vi "VI Interference Konfig.vi"() -> ()   [LabVIEW 2020, in "EPA 1065.lvlib" / "HovaCAL Interference verificaton.lvlib"]
uses:
  HovaCAL Interference verificaton.lvlib
  Tabelle.ctl
  TestKonfig.ctl
  TestKonfig H2O.ctl
  Modus.ctl
  Linearisierung V2/SpanEinstellungen/Einheit.ctl
  Linearisierung V2/Gasteiler/Stufen Tabelle 10 Stufen.ctl
  Linearisierung V2/Gasteiler/HovaCAL_Interface/Controls/Flow Einstellung.ctl
  Linearisierung V2/Gasteiler/HovaCAL_Interface/Controls/Temp Sollwerte Anzeige.ctl
  TestKonfig Interferents.ctl
  MFCAuswahl.ctl
  Seiten/System Einstellungen V2/Gasflasche Auswahl.ctl
  TestSetting.ctl
  Seiten/System Einstellungen V2/Analysatoren.ctl
  Visualisierungs Elemente/String - Ausgabefeld.ctl
  Visualisierungs Elemente/Button.ctl
  Tabelle Referenz.ctl
  Linearisierung V2/Gasteiler/HovaCAL_Interface/Controls/Pumpe Status Anzeige.ctl
  Linearisierung V2/Gasteiler/HovaCAL_Interface/Controls/Temp Ausgang Anzeige.ctl
  Linearisierung V2/Gasteiler/Gasteiler Fehler.ctl
  Linearisierung V2/Gasteiler/HovaCAL_Interface/Controls/Flow Anzeige.ctl
  Linearisierung V2/Gasteiler/HovaCAL_Interface/Controls/MFC Output plus Input Output Concentrations.ctl
  Sprachverwaltung/FGV Aktion Tabelle zerlegen.ctl
  Linearisierung V2/Gasteiler/Aktionen FGV Gasteiler Daten.ctl
  Aktion FGV Interference.ctl
  Aktion Test.ctl
  Allgemeine VIs/Aktion Test Status.ctl
  Allgemeine VIs/Aktion Wertaenderung Gasliste.ctl
  Linearisierung V2/GasteilerType.ctl
  Linearisierung V2/Gasteiler/HovaCAL_Interface/Kommunikation/Aktion_FGV_HovaCAL_Interface_GetData.ctl
  Linearisierung V2/Gasteiler/HovaCAL_Interface/Kommunikation/Aktion_FGV_HovaCAL_Interface_SetData.ctl
  Linearisierung V2/Aktion FGV Stoerungen sammeln und auswerten.ctl
  Linearisierung V2/LIN ErrorCluster.ctl
  Linearisierung V2/Gasteiler/Gasteiler Stufen.ctl
  Visualisierungs Elemente/String - Eingabefeld.ctl
  Aktion Index uebersetzten.ctl
  Allgemein/allgemeine Sub-VIs.lvlib
  Seiten/FT-IR/FT-IR.lvlib
  Sprachverwaltung/Sprachverwaltung.lvlib
  Linearisierung V2/Protokoll/Protokoll.lvlib
  EPA 1065.lvlib
  Seiten/System Einstellungen V2/System Einstellungen V2.lvlib
  Linearisierung V2/Gasteiler/HovaCAL_Interface/Kommunikation/Aktion_FGV_HovaCAL_Interface_Kommandos.ctl
  Linearisierung V2/Gasteiler/HovaCAL_Interface/Kommunikation/Kommunikation.lvlib
  Linearisierung V2/Gasteiler/Gasteiler.lvlib
  Linearisierung V2/Linearisierung v2.lvlib
  Linearisierung V2/Gasteiler/HovaCAL_Interface/HovaCAL_Interface.lvlib
  Linearisierung V2/SpanEinstellungen/SpanEinstellungen.lvlib
  Linearisierung V2/Gasteiler/HovaCAL_Interface/Controls/Controls.lvlib
panel:
  in  "Graph löschen":bool caption="Test Start"
  out "Graph PDF":waveform(dbl)[](graph) caption="Graph"
  in  "Daten löschen":bool caption="Test Start"
  in  "Save to file":bool caption="PDF erstellen"
  in  "Speichern":bool
  in  "Gasliste vergleichen":bool
  in  "Systemeinstellung":bool caption="Gasliste geändert"
  in  "Registerkarte":T1(tab)
  in  "TestSetting":T2
  in  "Abfragen":T4
  in  "Anforderung":T4
  in  "TestKonfig":T5={"TestKonfig H2O"={"Modus"=0, "Komponente:"=0, "Eingangs Konzentration:"=0.0, "Einheit"=enum."ppm", "Anzahl Stufen"=0.0, "Zeitdauer Stufen"=0.0, "Max Fehler"=1.0, "zusätzliche Zeitdauer Erster Punkt"=60.0, "Punkte umkehren"=FALSE, "Stufen Tabelle"=[], "HovaCAL Flow Input Cluster"={"HovaCAL Flow Input Cluster"=0.0}, "HovaCAL Temperature"=[]}, "TestKonfig Interferent"={"MFC1"=enum."MFC 1", "Eingangs Konzentration MFC1"=0.0, "Einheit MFC1 Eingang"=enum."ppm", "Ausgangs Konzentration MFC1"=0.0, "Einheit MFC1 Ausgang"=enum."ppm", "MFC2"=0, "Referenz-Interferent:"=0, "Gasflaschen Nr MFC2"="", "Accuracy MFC2"="", "Eingangs Konzentration MFC2"=0.0, "Einheit MFC2 Eingang"=enum."ppm", "Ausgangs Konzentration MFC2"=0.0, "Einheit MFC2 Ausgang"=enum."ppm", "MFC3"=1, "Kontroll-Interferent:"=0, "Gasflaschen Nr MFC3"="", "Accuracy MFC3"="", "Eingangs Konzentration MFC3"=0.0, "Einheit MFC3 Eingang"=enum."ppm", "Ausgangs Konzentration MFC3"=120.0, "Einheit MFC3 Ausgang"=enum."ppm", "Gasflasche MFC2"=0, "Gasflasche MFC3"=0}} {"TestKonfig H2O"."HovaCAL Temperature" format="%.2f"; "TestKonfig H2O"."HovaCAL Flow Input Cluster"."HovaCAL Flow Input Cluster" format="%.2f"; "TestKonfig H2O"."Eingangs Konzentration:" min=0.0; "TestKonfig H2O"."Komponente:" items=["H2O% (30) LP 191C", "H2Oppm (300000)"]; "TestKonfig H2O"."zusätzliche Zeitdauer Erster Punkt" min=60 step=1 format="%#_5g"; "TestKonfig H2O"."Zeitdauer Stufen" format="%#_5g"; "TestKonfig H2O"."Max Fehler" format="%#_5g"; "TestKonfig H2O"."Anzahl Stufen" format="%#_5g"; "TestKonfig H2O"."Modus" items=["Messen", "CG zu Entnahmestelle"]; "TestKonfig Interferent"."Gasflasche MFC3" items=["----"=10000, "IAG O2"=0, "IAG C2H2"=1, "IAG C2H4"=2, "IAG NH3 200"=3, "IAG NH3 2000"=4, "IAG NH3 3000"=5, "IAG CO 5%"=6, "IAG Propane 2%"=7, "IAG NO 1000"=8, "IAG SO2"=9, "IAG C3H6"=10, "IAG CO2"=11, "IAG CO"=12, "IAG N2O"=13, "IAG N2O 100"=14, "IAG NO2 1000"=15, "IAG NO2 100"=16, "IAG CH4"=17, "IAG Propane"=18, "Hansi"=19, "IAG MG"=20, "IAG NO 3000"=21, "CH42"=22]; "TestKonfig Interferent"."Gasflasche MFC2" items=["----"=10000, "IAG O2"=0, "IAG C2H2"=1, "IAG C2H4"=2, "IAG NH3 200"=3, "IAG NH3 2000"=4, "IAG NH3 3000"=5, "IAG CO 5%"=6, "IAG Propane 2%"=7, "IAG NO 1000"=8, "IAG SO2"=9, "IAG C3H6"=10, "IAG CO2"=11, "IAG CO"=12, "IAG N2O"=13, "IAG N2O 100"=14, "IAG NO2 1000"=15, "IAG NO2 100"=16, "IAG CH4"=17, "IAG Propane"=18, "Hansi"=19, "IAG MG"=20, "IAG NO 3000"=21, "CH42"=22]; "TestKonfig Interferent"."Eingangs Konzentration MFC1" min=0.0; "TestKonfig Interferent"."Ausgangs Konzentration MFC1" min=0.0; "TestKonfig Interferent"."MFC2" items=["MFC2", "MFC3"]; "TestKonfig Interferent"."MFC3" items=["MFC2", "MFC3"]; "TestKonfig Interferent"."Ausgangs Konzentration MFC3" min=0.0; "TestKonfig Interferent"."Eingangs Konzentration MFC3" min=0.0; "TestKonfig Interferent"."Ausgangs Konzentration MFC2" min=0.0; "TestKonfig Interferent"."Eingangs Konzentration MFC2" min=0.0; "TestKonfig Interferent"."Kontroll-Interferent:" items=["NO (3000) LP 191C", "NO2 (150) LP 191C (1of2)", "NO2 (2000) LP 191C (2of2)", "N2O (300) LP 191C (1of2)", "NH3 (300) LP 191C (1of2)", "NH3 (900,3000) LP 191C (2of2)", "HNCO (400) 191C", "H2O% (30) LP 191C", "Formaldehyde (70,500) LP 191C", "CO2 low% (4) LP 191C (2of2)", "CO2% (20) LP 191C (1of2)", "CO (700) LP 191C (1of3)", "CO% (1) LP 191C (2of3)", "Propylene (1000) LP 191C", "Aromatic HC C7 (500) LP 191C", "Ethylene (1000) LP 191C", "CH4 (250) LP 191C (1of2)", "CH4 (5000) LP 191C (2of2)", "Ethane (1000) LP 191C", "Acetylene (1000) LP 191C", "HNO2 (20) 191C", "MeOH (1000) 191C", "CO% (10) LP 191C (3of3)", "Formic Acid (100) 191C", "SO2 (500) LP 191C", "Acetaldehyde (1000) LP 191C", "COS (100) LP 191C", "1,3 butadiene (100) LP 191C", "Oil as Octane (200) LP 191C", "N2O (1000) LP 191C (2of2)", "Propane (200) LP 191C", "NO2 autorange (2000)", "CO autorange (100000)", "CH4 autorange (5000)", "NH3 autorange (3000)", "NOx autorange (3000)", "HCD (10000)", "NMHCD (10000)", "CO2% autorange (20)", "H2Oppm (300000)", "N2O autorange (1000)", "NMNEHCD (3000)", "Temp. Messzelle", "Druck Messzelle", "sBeam@2500", "Temp. HL zu FT-IR", "Temp. HL Extern SP1", "Austrittstemp. FT-IR", "Temp. Schaltschrank", "Konstant 0", "Konstant 50", "Konstant 100", "AK DUMMY"]; "TestKonfig Interferent"."Referenz-Interferent:" items=["NO (3000) LP 191C", "NO2 (150) LP 191C (1of2)", "NO2 (2000) LP 191C (2of2)", "N2O (300) LP 191C (1of2)", "NH3 (300) LP 191C (1of2)", "NH3 (900,3000) LP 191C (2of2)", "HNCO (400) 191C", "H2O% (30) LP 191C", "Formaldehyde (70,500) LP 191C", "CO2 low% (4) LP 191C (2of2)", "CO2% (20) LP 191C (1of2)", "CO (700) LP 191C (1of3)", "CO% (1) LP 191C (2of3)", "Propylene (1000) LP 191C", "Aromatic HC C7 (500) LP 191C", "Ethylene (1000) LP 191C", "CH4 (250) LP 191C (1of2)", "CH4 (5000) LP 191C (2of2)", "Ethane (1000) LP 191C", "Acetylene (1000) LP 191C", "HNO2 (20) 191C", "MeOH (1000) 191C", "CO% (10) LP 191C (3of3)", "Formic Acid (100) 191C", "SO2 (500) LP 191C", "Acetaldehyde (1000) LP 191C", "COS (100) LP 191C", "1,3 butadiene (100) LP 191C", "Oil as Octane (200) LP 191C", "N2O (1000) LP 191C (2of2)", "Propane (200) LP 191C", "NO2 autorange (2000)", "CO autorange (100000)", "CH4 autorange (5000)", "NH3 autorange (3000)", "NOx autorange (3000)", "HCD (10000)", "NMHCD (10000)", "CO2% autorange (20)", "H2Oppm (300000)", "N2O autorange (1000)", "NMNEHCD (3000)", "Temp. Messzelle", "Druck Messzelle", "sBeam@2500", "Temp. HL zu FT-IR", "Temp. HL Extern SP1", "Austrittstemp. FT-IR", "Temp. Schaltschrank", "Konstant 0", "Konstant 50", "Konstant 100", "AK DUMMY"]}
  out "%":dbl caption="Komponente max Fehler:"
  out "Kontrollinterferentwert":dbl caption="ppm"
  out "Referenzinterferentwert":dbl caption="ppm"
  out "Komponentenwert":dbl caption="%"
  out "Testdauer":dbl caption="verbleibende Testdauer" format="%.1f"
  out "Referenzwert:":T15
  out "Referenzwert":dbl caption="ppm"
  out "Interferent 2:":T15 caption="Kontroll-Interferent:"
  out "Interferent 1:":T15 caption="Referenz-Interferent:"
  in  "Abbrechen":bool caption="Test Start"
  out "Graph":waveform(dbl)[](graph)
  out "Status":string caption="Zustand"
  in  "Test Start":bool
  out "Komponente 1S:":T15 caption="Komponente:"
  out "Störung Kommunikation":bool
  out "Kontroll Interferent":T16 caption="Kontroll-Interferent"
  out "Referenz Interferent":T17 caption="Referenz-Interferent"
  out "Komponente":T16
  in  "Print to PDF":bool caption="PDF erstellen"
  out "Error":T18
  out "Cluster.Temp Cluster":T19 caption="Temp Ausgang"
  out "Cluster.PumpModeGeneral-Cluster":T20 caption="Pumpe Status"
  out "MFC Output":T21 caption="Fluss gesamt" {"Actual Flow" format="%.2f"}
  out "Pumpe":T22 {"water conc set" format="%.2f"; "water conc out" format="%.2f"}
  out "MFC1 Output":T23 caption="MFC1" {"Input Concentration" format="%.2f"; "Output Setpoint" format="%.2f"; "flow expected" format="%.2f"; "flow actual" format="%.2f"; "output concentration dry" format="%.2f"; "output concentration" format="%.2f"}
  out "MFC2 Output":T23 caption="MFC2" {"Input Concentration" format="%.2f"; "Output Setpoint" format="%.2f"; "flow expected" format="%.2f"; "flow actual" format="%.2f"; "output concentration dry" format="%.2f"; "output concentration" format="%.2f"}
  out "MFC3 Output":T23 caption="MFC3" {"Input Concentration" format="%.2f"; "Output Setpoint" format="%.2f"; "flow expected" format="%.2f"; "flow actual" format="%.2f"; "output concentration dry" format="%.2f"; "output concentration" format="%.2f"}
  # "HovaCAL Querempfindlichkeitsnachweis"
  # "Allgemeine Einstellungen"
  # "Protokoll Einstellungen"
  # "Wasser"
  # "Stickstoff"
  # "Referenz-Interferent"
  # "Kontroll-Interferent"
  # "sec"
  # "%"
  # "sec"
  # "Test"
  # "sec"
  # "Ergebnis"
  # "%"
  # "%"
  # "l/min"
  # "l/min"
  # "l/min"
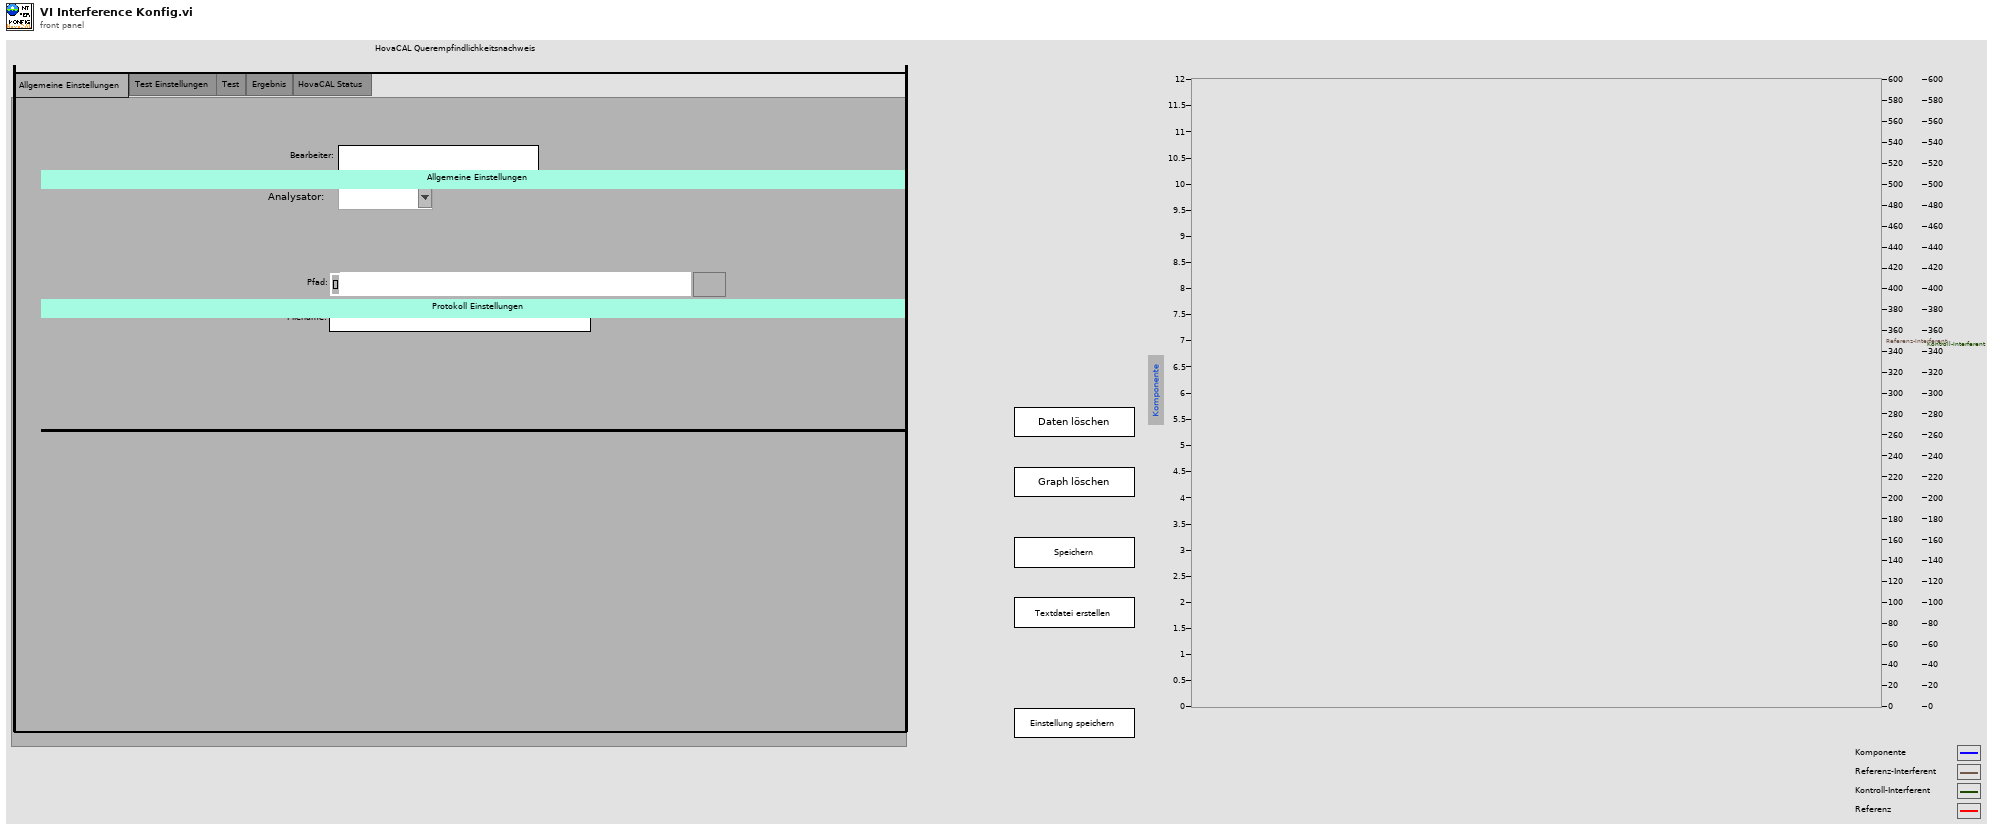
[diagram p1: front panel]
types:
  T1 = enum32{"General Settings", "Test Settings", "Test", "Result", "HovaCAL Status"}
  T2 = typedef "EPA 1065.lvlib/HovaCAL Interference verificaton.lvlib/TestSetting.ctl" = cluster{"Bearbeiter:":string, "Pfad:":path, "Textname:":string, "Analysator":T3}
  T3 = typedef "System Einstellungen V2.lvlib/Analysatoren.ctl" = string
  T4 = typedef "Button.ctl" = bool
  T5 = typedef "EPA 1065.lvlib/HovaCAL Interference verificaton.lvlib/TestKonfig.ctl" = cluster{"TestKonfig H2O":T6, "TestKonfig Interferent":T12}
  T6 = typedef "EPA 1065.lvlib/HovaCAL Interference verificaton.lvlib/TestKonfig H2O.ctl" = cluster{"Modus":T7, "Komponente:":u16, "Eingangs Konzentration:":dbl, "Einheit":T8, "Anzahl Stufen":sgl, "Zeitdauer Stufen":sgl, "Max Fehler":sgl, "zusätzliche Zeitdauer Erster Punkt":sgl, "Punkte umkehren":bool, "Stufen Tabelle":T9, "HovaCAL Flow Input Cluster":T10, "HovaCAL Temperature":T11}
  T7 = typedef "EPA 1065.lvlib/HovaCAL Interference verificaton.lvlib/Modus.ctl" = u16
  T8 = typedef "Linearisierung v2.lvlib/SpanEinstellungen.lvlib/Einheit.ctl" = enum16{"ppm", "%"}
  T9 = typedef "Linearisierung v2.lvlib/Gasteiler.lvlib/Stufen Tabelle 10 Stufen.ctl" = string[][]
  T10 = typedef "Linearisierung v2.lvlib/Gasteiler.lvlib/HovaCAL_Interface.lvlib/Controls.lvlib/Flow Einstellung.ctl" = cluster{"HovaCAL Flow Input Cluster":dbl}
  T11 = typedef "Linearisierung v2.lvlib/Gasteiler.lvlib/HovaCAL_Interface.lvlib/Controls.lvlib/Temp Sollwerte Anzeige.ctl" = dbl[]
  T12 = typedef "EPA 1065.lvlib/HovaCAL Interference verificaton.lvlib/TestKonfig Interferents.ctl" = cluster{"MFC1":enum16{"MFC 1"}, "Eingangs Konzentration MFC1":dbl, "Einheit MFC1 Eingang":T8, "Ausgangs Konzentration MFC1":dbl, "Einheit MFC1 Ausgang":T8, "MFC2":T13, "Referenz-Interferent:":u16, "Gasflaschen Nr MFC2":string, "Accuracy MFC2":string, "Eingangs Konzentration MFC2":dbl, "Einheit MFC2 Eingang":T8, "Ausgangs Konzentration MFC2":dbl, "Einheit MFC2 Ausgang":T8, "MFC3":T13, "Kontroll-Interferent:":u16, "Gasflaschen Nr MFC3":string, "Accuracy MFC3":string, "Eingangs Konzentration MFC3":dbl, "Einheit MFC3 Eingang":T8, "Ausgangs Konzentration MFC3":dbl, "Einheit MFC3 Ausgang":T8, "Gasflasche MFC2":T14, "Gasflasche MFC3":T14}
  T13 = typedef "EPA 1065.lvlib/HovaCAL Interference verificaton.lvlib/MFCAuswahl.ctl" = u16
  T14 = typedef "System Einstellungen V2.lvlib/Gasflasche Auswahl.ctl" = u16
  T15 = typedef "String - Ausgabefeld.ctl" = string
  T16 = typedef "EPA 1065.lvlib/HovaCAL Interference verificaton.lvlib/Tabelle.ctl" = string[][]
  T17 = typedef "EPA 1065.lvlib/HovaCAL Interference verificaton.lvlib/Tabelle Referenz.ctl" = string[][]
  T18 = typedef "Linearisierung v2.lvlib/Gasteiler.lvlib/Gasteiler Fehler.ctl" = cluster{"Pressure carrier gas":bool, "Pressure diluted gas":bool, "Outlet Pressure":bool, "SNOX before SAIR":bool}
  T19 = typedef "Linearisierung v2.lvlib/Gasteiler.lvlib/HovaCAL_Interface.lvlib/Controls.lvlib/Temp Ausgang Anzeige.ctl" = cluster{"temp 2":dbl, "temp":dbl, "humidity":dbl}[]
  T20 = typedef "Linearisierung v2.lvlib/Gasteiler.lvlib/HovaCAL_Interface.lvlib/Controls.lvlib/Pumpe Status Anzeige.ctl" = cluster{"running?":bool, "Speed":dbl[]}
  T21 = typedef "Linearisierung v2.lvlib/Gasteiler.lvlib/HovaCAL_Interface.lvlib/Controls.lvlib/Flow Anzeige.ctl" = cluster{"Actual Flow":dbl}
  T22 = cluster{"water conc set":dbl, "water conc out":dbl}
  T23 = typedef "Linearisierung v2.lvlib/Gasteiler.lvlib/HovaCAL_Interface.lvlib/Controls.lvlib/MFC Output plus Input Output Concentrations.ctl" = cluster{"Input Concentration":dbl, "Output Setpoint":dbl, "output concentration":dbl, "output concentration dry":dbl, "flow actual":dbl, "flow expected":dbl}
  T24 = typedef "EPA 1065.lvlib/HovaCAL Interference verificaton.lvlib/Aktion Test.ctl" = enum16{"Lesen", "ini", "ini-Warten-Stabil", "Warten-Stabil", "ini-warten-aufzeichnen", "Warten-Aufzeichnen", "aufzeichnen", "fertig", "spülen", "abbrechen"}
  T25 = typedef "EPA 1065.lvlib/HovaCAL Interference verificaton.lvlib/Aktion FGV Interference.ctl" = enum16{"Lesen", "TestKonfig", "TestSetting", "Einheiten", "Ergebnis", "Laden", "Tabelle", "Speichern", "löschen"}
  T26 = typedef "Linearisierung v2.lvlib/Gasteiler.lvlib/Aktionen FGV Gasteiler Daten.ctl" = enum16{"lesen", "Gasteiler Daten", "Seriellen Param.", "MB-Endwert", "laden", "speichern", "Anforderung", "TCP", "Aufzeichnung Start"}
  T27 = typedef "Sprachverwaltung.lvlib/FGV Aktion Tabelle zerlegen.ctl" = enum16{"laden", "vereinzeln", "speichern"}
  T28 = typedef "EPA 1065.lvlib/HovaCAL Interference verificaton.lvlib/Komponenten.ctl" = cluster{"Komponente":T15, "Komponente Index":i32, "Referenz Interferent":T15, "Refernz Interferent Index":i32, "Kontroll Interferent":T15, "Kontroll Interferent Index":i32, "Einheit Komponente":string, "Einheit Refernz Interferrent":string, "Einheit Kontroll Interferrent":string}
  T29 = typedef "Linearisierung v2.lvlib/Gasteiler.lvlib/HovaCAL_Interface.lvlib/Kommunikation.lvlib/Aktion_FGV_HovaCAL_Interface_GetData.ctl" = enum16{"lesen", "SystemInfo", "MFC Info", "actual Values", "Limits", "first contact", "reset after read"}
  T30 = enum8{"Enabled", "Disabled", "Disabled and Grayed Out"}
  T31 = typedef "EPA 1065.lvlib/Aktion Wertaenderung Gasliste.ctl" = enum16{"Init", "lesen", "Gasliste geändert", "ARN inaktiv", "LEAK inaktiv", "Interference 366 inaktiv", "T90 inaktiv", "Interference 375 inaktiv", "Chiller inaktiv", "FID O2 inaktiv", "FID Opti inaktiv", "Drift inaktiv", "Pre Test inaktiv", "LinV2 inaktiv", "HovaCAL Interference inaktiv"}
  T32 = typedef "EPA 1065.lvlib/Aktion Test Status.ctl" = enum16{"init", "lesen", "prüfen", "Interference 366", "Interference 375", "Chiller läuft", "Drift läuft", "Pre Test läuft", "FID Optimization läuft", "FID Interference läuft", "HovaCAL Interference", "LinV2"}
  T33 = typedef "Linearisierung v2.lvlib/Gasteiler.lvlib/HovaCAL_Interface.lvlib/Kommunikation.lvlib/Aktion_FGV_HovaCAL_Interface_SetData.ctl" = enum16{"lesen", "Konzentrationen", "Pumpen Parameter", "Pumpe Konzentration", "Pumpe run", "Temperaturen", "Fluss", "Limits", "init"}
  T34 = typedef "Linearisierung v2.lvlib/Gasteiler.lvlib/HovaCAL_Interface.lvlib/Kommunikation.lvlib/Aktion_FGV_HovaCAL_Interface_Kommandos.ctl" = enum16{"lesen", "verarbeiten", "hinzufügen", "on top", "init", "sammeln", "freigeben", "connected"}
  T35 = enum32{"General Settings", "Test Settings", "Test", "Result"}
  T36 = typedef "String - Eingabefeld.ctl" = string
  T37 = typedef "Linearisierung v2.lvlib/LIN ErrorCluster.ctl" = cluster{"Störung Kommunikation":bool, "Pressure carrier gas":bool, "Pressure diluted gas":bool, "Outlet Pressure":bool, "SNOX before SAIR":bool, "Störung Gasteiler":bool}
  T38 = typedef "Linearisierung v2.lvlib/Aktion FGV Stoerungen sammeln und auswerten.ctl" = enum16{"init", "lesen", "error", "prüfen", "reset error", "abbrechen", "fortsetzen", "neustart", "Bedientasten reset"}
  T39 = typedef "EPA 1065.lvlib/HovaCAL Interference verificaton.lvlib/Aktion Index uebersetzten.ctl" = enum16{"lesen", "schreiben", "auswerten", "Referenzwert", "KompIndex", "RefInterferIndex", "KontrInterfIndex"}
  T40 = enum16{"open", "replace", "create", "open or create", "replace or create", "replace or create with confirmation"}
  T41 = cluster{"first contact in":bool, "first actual values in ":bool}
  T42 = typedef "Linearisierung v2.lvlib/GasteilerType.ctl" = u16
  T43 = typedef "EPA 1065.lvlib/Aktive Tests Cluster.ctl" = cluster{"ANR läuft":bool, "T90 läuft":bool, "Leak läuft":bool, "Interference 366 läuft":bool, "Interference 375 läuft":bool, "Chiller läuft":bool, "FID Interference läuft":bool, "FID optimization läuft":bool, "Drift läuft":bool, "Pre-test läuft":bool, "HovaCAL Interference läuft":bool, "LinV2 läuft":bool}
  T44 = typedef "LVDateTimeRec.ctl" = cluster{"Sekundenbruchteil":dbl, "Sekunde":i32, "Minute":i32, "Stunde":i32, "Tag des Monats":i32, "Monat":i32, "Jahr":i32, "Wochentag":i32, "Tag des Jahres":i32, "DST":i32}
  T45 = cluster{"temp 2":dbl, "temp":dbl, "humidity":dbl}[]
  T46 = typedef "Linearisierung v2.lvlib/Gasteiler.lvlib/HovaCAL_Interface.lvlib/Controls.lvlib/Info Cluster.ctl" = cluster{"device":string, "version":string, "number of mfc":i32, "number of pumps":i32, "number of temp controllers":i32, "number of mfs":i32, "number of balances":i32}
  T47 = cluster{"HovaCAL Temperature":refnum<vi>, "Cluster.Temp Cluster":refnum<vi>, "Cluster.PumpModeGeneral-Cluster":refnum<vi>, refnum<vi>[]}
  T48 = typedef "Linearisierung v2.lvlib/Gasteiler.lvlib/Gasteiler Stufen.ctl" = u16
  T49 = typedef "Linearisierung v2.lvlib/Gasteiler.lvlib/Gasteiler Daten.ctl" = cluster{"Gasteiler":T36, "Gasteiler Stufen":T48, "Gasteiler Type":T42, "Konfig Gasteiler":T50, "Gasteiler Span Eingänge":u16}
  T50 = typedef "System Einstellungen V2.lvlib/Gasteiler Auswahl.ctl" = u16
  T51 = cluster{"Komponente:":u16, "Eingangs Konzentration:":dbl}[]
  T52 = cluster{"Komponente:":u16, "Eingangs Konzentration:":dbl}
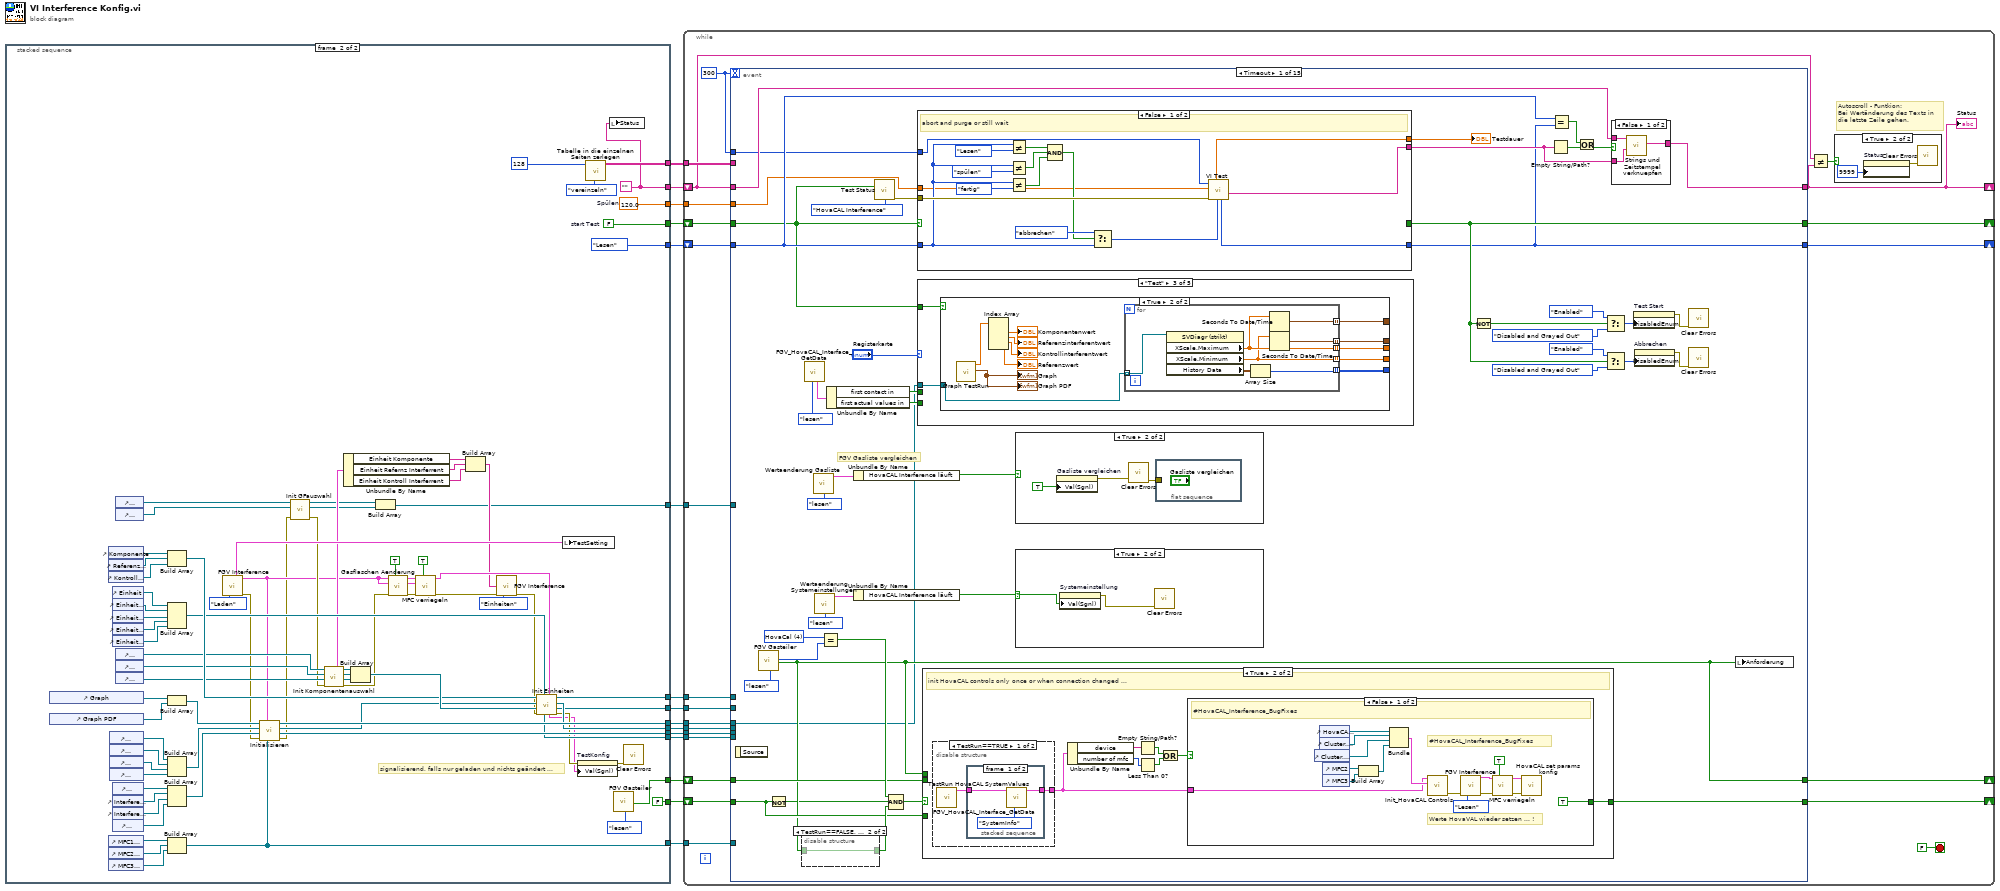
[diagram p0: block diagram]
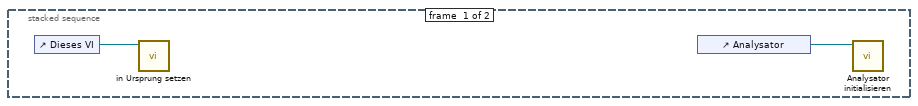
[diagram p2: hidden frame]
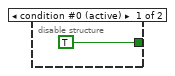
[diagram p3: hidden frame]
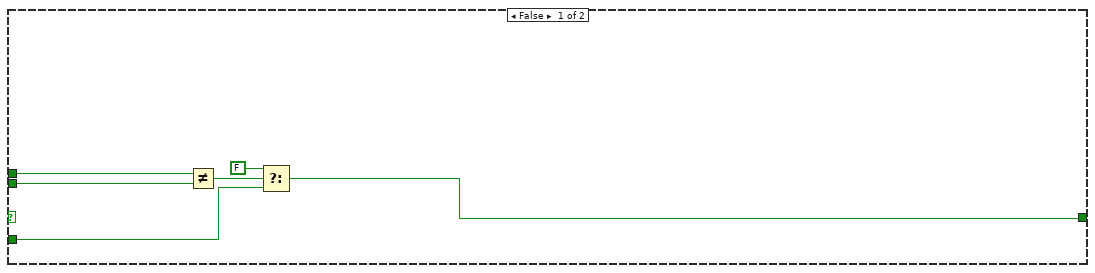
[diagram p4: hidden frame]
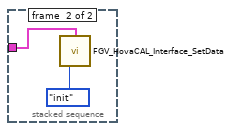
[diagram p6: hidden frame]
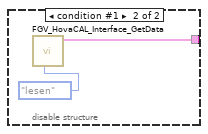
[diagram p7: hidden frame]
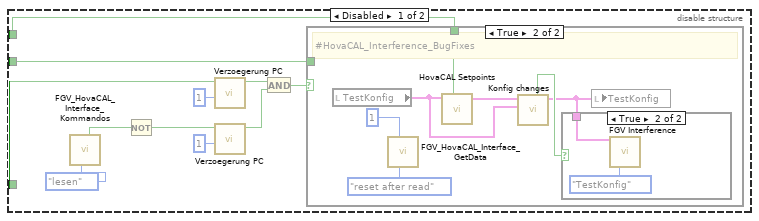
[diagram p12: hidden frame]
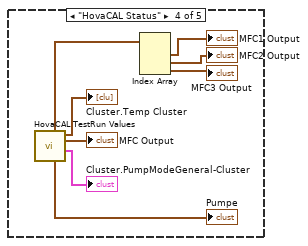
[diagram p16: hidden frame]
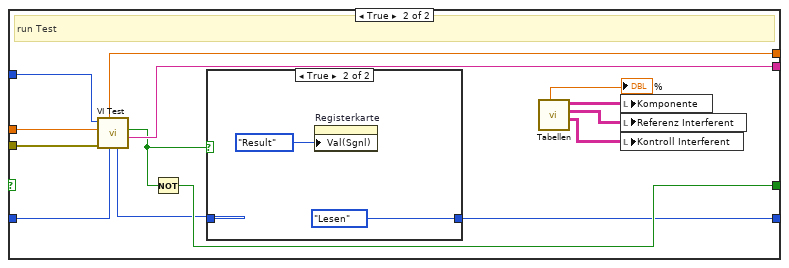
[diagram p18: hidden frame]
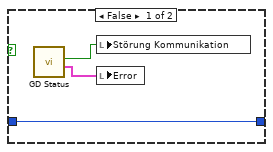
[diagram p19: hidden frame]
diagram:
  n1 = stacked-sequence {
    tunnel: [_ w97] -> w15
    tunnel: [_ w90] -> w14
    tunnel: [_ w87] -> w13
    tunnel: [_ w80] -> w12
    tunnel: [_ w86] -> w11
    tunnel: [_ w79] -> w10
    tunnel: [_ FALSE] -> w9
    tunnel: [_ w62] -> w8
    tunnel: [_ w69] -> w7
    tunnel: [_ w60] -> w6
    tunnel: [_ Aktion_Test."Lesen" ("Aktion")] -> w5
    tunnel: [_ w35] -> w4
    tunnel: [_ w26] -> w3
    tunnel: [_ w19] -> w2
    tunnel: [_ w18] -> w1
    frame #0 {
      n2 = control-ref of="Dieses VI"() -> (w16:refnum<vi>)
      n3 = call "in Ursprung setzen.vi"("VI Referenz"=w16) -> ()  [unwired: 10 in, 1 out]
      n4 = control-ref of="Analysator"() -> (w17:refnum<vi>)
      n5 = call "Analysator initialisieren.vi"("Referenz Analysator"=w17) -> ()  [unwired: 9 in, 2 out]
    }
    frame #1 {
      w18 = 120.0  # Spülen
      w35 = ""
      w90 = FALSE  # start Test
      # "signalisierend, falls nur geladen und nichts geändert ..."
      n6 = control-ref of="Graph"() -> (w88:refnum<vi>)
      n7 = control-ref of="Graph PDF"() -> (w75:refnum<vi>)
      n8 = control-ref of="Komponente"() -> (w73:refnum<vi>)
      n9 = control-ref of="Referenz Interferent"() -> (w72:refnum<vi>)
      n10 = control-ref of="Kontroll Interferent"() -> (w71:refnum<vi>)
      n11 = control-ref of="MFC1 Output"() -> (w22:refnum<vi>)
      n12 = control-ref of="MFC2 Output"() -> (w21:refnum<vi>)
      n13 = control-ref of="MFC3 Output"() -> (w20:refnum<vi>)
      n14 = control-ref of="Komponentenwert"() -> (w32:refnum<vi>)
      n15 = control-ref of="Referenzinterferentwert"() -> (w33:refnum<vi>)
      n16 = control-ref of="Kontrollinterferentwert"() -> (w34:refnum<vi>)
      n17 = control-ref of="Referenzwert"() -> (w77:refnum<vi>)
      n18 = control-ref of="Einheit"() -> (w68:refnum<vi>)
      n19 = control-ref of="Einheit MFC2 Eingang"() -> (w67:refnum<vi>)
      n20 = control-ref of="Einheit MFC2 Ausgang"() -> (w66:refnum<vi>)
      n21 = control-ref of="Einheit MFC3 Eingang"() -> (w65:refnum<vi>)
      n22 = control-ref of="Einheit MFC3 Ausgang"() -> (w64:refnum<vi>)
      n23 = control-ref of="Komponente 1S:"() -> (w89:refnum<vi>)
      n24 = control-ref of="Interferent 1:"() -> (w94:refnum<vi>)
      n25 = control-ref of="Interferent 2:"() -> (w95:refnum<vi>)
      n26 = control-ref of="Referenzwert:"() -> (w78:refnum<vi>)
      n27 = control-ref of="Gasflasche MFC2"() -> (w31:refnum<vi>)
      n28 = control-ref of="Gasflasche MFC3"() -> (w30:refnum<vi>)
      n29 = control-ref of="Komponente:"() -> (w49:refnum<vi>)
      n30 = control-ref of="Referenz-Interferent:"() -> (w48:refnum<vi>)
      n31 = control-ref of="Kontroll-Interferent:"() -> (w47:refnum<vi>)
      n32 = Build Array(w73, w72, w71) -> (w63:refnum<vi>[])
      n33 = Build Array(w68, w67, w66, w65, w64) -> (w61:refnum<vi>[])
      n34 = Build Array(w88, w75) -> (w76:refnum<vi>[])
      n35 = Build Array(w32, w33, w34, w77) -> (w93:refnum<vi>[])
      n36 = Build Array(w89, w94, w95, w78) -> (w92:refnum<vi>[])
      n37 = Build Array(w22, w21, w20) -> (w19:refnum<vi>[])
      n38 = call "FGV Interference.vi"("Aktion FGV Interference"=Aktion_FGV_Interference."Laden") -> ("TestSetting"=w58:T2, "TestKonfig"=w25:T5, "error out"=w24:errorcluster)  [unwired: 9 in, 3 out]
      n39 = call "Initialisieren.vi"("MFC Cluster Array"=w19, "TestKonfig (Eingang)"=w25, "Fehler (Eingang)"=w24, "Strings Array in"=w92, "Ergebnis  Array in"=w93, "Signalverlaufsdiagramm (Eingang)"=w76) -> ("Fehler (Ausgang)"=w23:errorcluster, "Strings Array out"=w86:refnum<vi>[], "Ergenis Arry out"=w81:refnum<vi>[], "Signalverlaufsdiagramm (Ausgang)"=w87:refnum<vi>[])  [unwired: 2 in]
      n40 = call "Init GFauswahl.vi"("Fehler (Eingang, kein Fehler)"=w23, "GF MFC3 (Eingang)"=w30, "GF MFC2 (Eingang)"=w31) -> ("Fehler (Ausgang)"=w29:errorcluster, "GF MFC3 (Ausgang)"=w27:refnum<vi>, "GF MFC2 (Ausgang)"=w28:refnum<vi>)  [unwired: 6 in]
      n41 = call "Init Komponentenauswahl.vi"("Fehler (Eingang, kein Fehler)"=w29, "Kontroll-Interferent: (Eingang)"=w47, "Refernz-Interferent: (Eingang)"=w48, "Komponente: (Eingang)"=w49) -> ("Fehler (Ausgang)"=w40:errorcluster, "Kontroll-Interferent: (Ausgang)"=w83:refnum<vi>, "Refernz-Interferent:  (Ausgang)"=w84:refnum<vi>, "Komponente: (Ausgang)"=w85:refnum<vi>, "Komponenten"=w41:T28)  [unwired: 3 in]
      n42 = Unbundle By Name(w41) -> ("Einheit Komponente"=w45:string, "Einheit Refernz Interferrent"=w44:string, "Einheit Kontroll Interferrent"=w43:string)
      n43 = Build Array(w85, w84, w83) -> (w82:refnum<vi>[])
      n44 = Build Array(w28, w27) -> (w26:refnum<vi>[])
      n45 = call "Gasflaschen Aenderung.vi"("init"=TRUE, "Fehler (Eingang, kein Fehler)"=w40, "TestKonfig alt"=w25, "TestKonfig (Eingang)"=w25) -> ("Fehler (Ausgang)"=w51:errorcluster, "TestKonfig alt out"=w52:T5, "TestKonfig (Ausgang)"=w53:T5)  [unwired: 5 in]
      n46 = call "MFC verriegeln.vi"("init"=TRUE, "Fehler (Eingang, kein Fehler)"=w51, "TestKonfig alt (Eingang)"=w52, "TestKonfig (Eingang)"=w53) -> ("Fehler (Ausgang)"=w39:errorcluster, "TestKonfig (Ausgang)"=w50:T5)  [unwired: 5 in, 1 out]
      n47 = Build Array(w45, w44, w43) -> (w42:string[])
      n48 = call "FGV Interference.vi"("Einheiten"=w42, "error in (no error)"=w39, "Aktion FGV Interference"=Aktion_FGV_Interference."Einheiten") -> ("error out"=w38:errorcluster)  [unwired: 7 in, 5 out]
      n49 = call "Init Einheiten.vi"("TestKonfig (Eingang)"=w50, "Units Array in"=w61, "Fehler (Eingang, kein Fehler)"=w38, "Komp. Auswahl Array"=w82, "Ergebnis Array in"=w81, "Table Array in"=w63) -> ("Fehler (Ausgang)"=w55:errorcluster, "Komp. Auswahl Array out"=w79:refnum<vi>[], "Ergebnis Array out"=w80:refnum<vi>[], "Table Array out"=w62:refnum<vi>[], "TestKonfig (Ausgang)"=w37:T5, "Units Array out"=w60:refnum<vi>[])
      n50 = local write "TestSetting"(w58) -> ()
      n51 = property on="TestKonfig" class="Cluster (strikt)"(error in=w55, "Val(Sgnl)"=w37) -> (error out=w59:errorcluster)  [unwired: 1 in, 1 out]
      n52 = call "Tabelle in die einzelnen Seiten zerlegen.vi"("Aktion"=FGV_Aktion_Tabelle_zerlegen."vereinzeln", "Index (Seite)"=128) -> ("Sprachliste"=w97:string[][])  [unwired: 7 in, 2 out]
      n53 = local write "Status"(w35) -> ()
      n54 = call "FGV Gasteiler.vi"("Aktionen"=Aktionen_FGV_Gasteiler_Daten."lesen") -> ("Anforderung"=w69:bool)  [unwired: 11 in, 7 out]
      n55 = call <vilib>:"Clear Errors.vi"("error in (no error)"=w59) -> ()  [unwired: 5 in, 2 out]
    }
  }
  n56 = while {
    shift-right: [w118] -> _
    shift-left: w14 -> [w119]
    shift-right: [w114] -> _
    shift-left: w4 -> [w116]
    tunnel: w15 -> [w117]
    shift-right: [w113] -> _
    shift-left: w5 -> [w112]
    tunnel: w13 -> [w111]
    tunnel: w12 -> [w110]
    tunnel: w11 -> [w109]
    tunnel: w10 -> [w108]
    shift-right: [w106] -> _
    shift-left: w9 -> [w107]
    tunnel: w8 -> [w105]
    shift-right: [w104] -> _
    shift-left: w7 -> [w103]
    tunnel: w6 -> [w102]
    tunnel: w3 -> [w100]
    tunnel: w2 -> [w99]
    tunnel: w1 -> [w98]
    stop <- FALSE stop-if-true
    w101 = 300
    # "Autoscroll - Funtkion:\nBei Wertänderung des Texts in \ndie letzte Zeile gehen."
    n57 = event shown="[0] Timeout" {
      selector: _ -> [_ _ _ _ _ _ _ _ _ _ _ _ _ _ _]
      dyn-events: _ -> [_ _ _ _ _ _ _ _ _ _ _ _ _ _ _]
      timeout: w101 -> [_ _ _ _ _ _ _ _ _ _ _ _ _ _ _]
      tunnel: [w165 w331 w355 w365 w385 w439 w478 w481 w558 w569 w592 w605 w628 w636 w642] -> w114
      tunnel: w116 -> [w164 w331 w355 w365 w385 w439 w478 _ w557 w569 w592 w605 w628 w636 w642]
      tunnel: w119 -> [w127 w330 w356 w362 w386 w441 w477 _ _ w571 w591 w604 w630 w638 w643]
      tunnel: [w145 w330 w356 w361 w386 w441 w477 w493 FALSE w571 w591 w604 w630 w638 w643] -> w118
      tunnel: w117 -> [_ _ _ w359 _ _ w443 w489 w554 _ _ _ _ _ _]
      tunnel: [w131 w329 w357 w364 w387 w440 w476 w491 w556 w570 w590 w603 w629 w637 w644] -> w113
      tunnel: w112 -> [w130 w329 w357 w364 w387 w440 w476 w490 w556 w570 w590 w603 w629 w637 w644]
      tunnel: w111 -> [w121 _ _ _ _ w426 _ w483 _ _ w578 _ _ w634 _]
      tunnel: w110 -> [_ _ _ _ _ w438 w451 w482 _ _ _ _ _ w633 _]
      tunnel: w109 -> [_ _ _ _ _ w437 _ _ _ _ _ _ _ _ _]
      tunnel: w108 -> [_ _ _ _ _ w436 w450 _ _ _ _ _ _ _ _]
      tunnel: w107 -> [w136 _ w332 w358 w381 w390 w442 w480 w547 w565 w572 w601 w626 w632 w639]
      tunnel: [w138 FALSE ("t") w332 w358 w381 w390 w442 w480 w547 w565 w572 w601 w626 w632 w639] -> w106
      tunnel: w105 -> [_ _ _ _ _ w415 w452 _ _ _ _ _ _ _ _]
      tunnel: [w134 w305 w354 w363 w382 w417 w475 w484 w548 w566 w576 w602 w627 w635 w641] -> w104
      tunnel: w103 -> [w135 w305 w354 w363 w382 w417 w475 w484 w548 w566 w576 w602 w627 w635 w641]
      tunnel: w102 -> [_ _ _ _ _ w416 w453 _ _ _ _ _ _ _ _]
      tunnel: w101 -> [w128 _ _ _ _ _ _ _ _ _ _ _ _ _ _]
      tunnel: w100 -> [_ _ _ w360 _ _ _ _ _ _ _ _ _ _ _]
      tunnel: w99 -> [_ _ _ _ _ w392 _ _ _ _ _ _ _ _ _]
      tunnel: w98 -> [w122 _ _ _ _ _ _ w479 _ _ _ _ _ _ _]
      event Timeout {
        w142 = T42 4 items=["LNI", "Analog-Display", "AVL GDU", "Horiba GDC", "HovaCal", "Horiba SGD 710C"] ("x")
        # "FGV Gasliste vergleichen"
        n58 = event-data() -> ()  [unwired: 1 in, 1 out]
        n59 = call "FGV Gasteiler.vi"("Aktionen"=Aktionen_FGV_Gasteiler_Daten."lesen") -> ("Gasteiler Type"=w141:T42, "Anforderung"=w134:bool)  [unwired: 11 in, 6 out]
        n60 = Not(x=w136) -> (.not. x?=w129:bool)
        n61 = disable-structure shown="TestRun==FALSE, Standard" {
          disable-tunnel: [TRUE w169] -> w137
          disable-tunnel: w134 -> [_ w169]
          frame condition #0 (active) {
          }
          frame condition #1 {
          }
        }
        n62 = call "FGV_HovaCAL_Interface_GetData.vi"("Aktion"=Aktion_FGV_HovaCAL_Interface_GetData."lesen") -> ("first flags out"=w126:T41)  [unwired: 6 in, 4 out]
        n63 = call "Wertaenderung Gasliste.vi"("Aktion"=Aktion_Wertaenderung_Gasliste."lesen") -> ("Tests"=w160:T43)  [unwired: 13 in, 1 out]
        n64 = call "Wertaenderung Systemeinstellungen.vi"("Aktion"=Aktion_Wertaenderung_Gasliste."lesen") -> ("Tests"=w156:T43)  [unwired: 13 in, 1 out]
        n65 = Equal?(x=w142, y=w141) -> (x = y?=w139:bool)
        n66 = Unbundle By Name(w126) -> ("first contact in"=w123:bool, "first actual values in"=w124:bool)
        n67 = Unbundle By Name(w160) -> ("HovaCAL Interference läuft"=w159:bool)
        n68 = Unbundle By Name(w156) -> ("HovaCAL Interference läuft"=w157:bool)
        n69 = call "Test Status.vi"("HovaCAL Interference läuft"=w127, "Aktion"=Aktion_Test_Status."HovaCAL Interference") -> ("error out"=w155:errorcluster)  [unwired: 10 in, 3 out]
        n70 = Compound Arithmetic op=AND ("Mehrfacharithmetik")(w139, w129, w137) -> (w140:bool)
        n71 = case shown="False" w127 {
          tunnel: [w279 w294] -> w166
          tunnel: w130 -> [w270 w293]
          tunnel: [_ w292] -> w145
          tunnel: [w278 w291] -> w154
          tunnel: w155 -> [w274 w289]
          tunnel: [w266 w287] -> w131
          tunnel: w128 -> [w267 w283]
          tunnel: w122 -> [w265 w281]
          frame False {
            # "abort and purge or still wait"
            n72 = Not Equal?(x=w270, y=Aktion_Test."Lesen" ("Aktion")) -> (x != y?=w277:bool)
            n73 = Not Equal?(x=w270, y=Aktion_Test."spülen" ("Aktion")) -> (x != y?=w269:bool)
            n74 = Not Equal?(x=w270, y=Aktion_Test."fertig" ("Aktion")) -> (x != y?=w268:bool)
            n75 = Compound Arithmetic op=AND ("Mehrfacharithmetik")(w277, w269, w268) -> (w271:bool)
            n76 = Select(t=Aktion_Test."abbrechen", s=w271, f=w270) -> (s? t:f=w276:T24)
            n77 = call "VI Test.vi"("Aktion"=w276, "error in (no error)"=w274, "Spülen"=w265, "KommLoopTimer"=w267) -> ("Status Test"=w279:string, "Aktion"=w266:T24, "Warten"=w278:dbl)  [unwired: 2 in, 3 out]
          }
          frame True {
            # "run Test"
            n78 = call "VI Test.vi"("Aktion"=w293, "error in (no error)"=w289, "Spülen"=w281, "KommLoopTimer"=w283) -> ("Status Test"=w294:string, "Fertig"=w290:bool, "Aktion"=w288:T24, "Warten"=w291:dbl)  [unwired: 2 in, 2 out]
            n79 = Not(x=w290) -> (.not. x?=w292:bool)
            n80 = case shown="True" w290 {
              tunnel: w288 -> [w297 _]
              tunnel: [w297 Aktion_Test."Lesen" ("Aktion")] -> w287
              frame False {
                n81 = call "GD Status.vi"() -> ("Error"=w295:T18, "Störung"=w296:bool)  [unwired: 9 in, 1 out]
                n82 = local write "Störung Kommunikation"(w296) -> ()
                n83 = local write "Error"(w295) -> ()
              }
              frame True {
                n84 = property on="Registerkarte" class="RKElem (strikt)"("Val(Sgnl)"=T35."Result" ("Registerkarte")) -> ()  [unwired: 2 in, 2 out]
              }
            }
            n85 = call "Tabellen.vi"() -> ("Tabelle Kontroll Interferent"=w285:string[][], "Tabbelle Referenz Interferent"=w284:string[][], "Tabelle Komponente"=w286:string[][], "Max. Fehler Komponente"=→"%":dbl)  [unwired: 5 in, 3 out]
            n86 = local write "Komponente"(w286) -> ()
            n87 = local write "Referenz Interferent"(w284) -> ()
            n88 = local write "Kontroll Interferent"(w285) -> ()
          }
        }
        "Testdauer" <- w154
        n89 = case shown="\"Test\"" "Registerkarte" {
          tunnel: w127 -> [_ w215 w237 _ _]
          tunnel: w123 -> [_ w214 _ _ _]
          tunnel: w124 -> [_ w213 _ _ _]
          tunnel: w121 -> [_ _ w236 _ _]
          frame "General Settings", Default {
          }
          frame "Test Settings" {
            n90 = disable-structure shown="Aktiviert" {
              disable-tunnel: w215 -> [w218 _]
              disable-tunnel: w214 -> [w217 _]
              disable-tunnel: w213 -> [w216 _]
              frame Disabled {
                n91 = call "FGV_HovaCAL_Interface_Kommandos.vi"("Aktion"=Aktion_FGV_HovaCAL_Interface_Kommandos."lesen") -> ("gesammelt ?"=w224:bool)  [unwired: 4 in, 5 out]
                n92 = Not(x=w224) -> (.not. x?=w225:bool)
                n93 = call "Verzoegerung PC.vi"("sec"=u16 1, "Startsignal"=w216) -> ("Zeit abgelaufen?"=w223:bool)  [unwired: 8 in, 1 out]
                n94 = call "Verzoegerung PC.vi"("sec"=u16 1, "Startsignal"=w225) -> ("Zeit abgelaufen?"=w226:bool)  [unwired: 8 in, 1 out]
                n95 = And(x=w223, y=w226) -> (x .and. y?=w219:bool)
                n96 = case shown="True" w219 {
                  tunnel: w217 -> [_ _]
                  tunnel: w218 -> [_ w229]
                  frame False {
                  }
                  frame True {
                    # "#HovaCAL_Interference_BugFixes"
                    n97 = local read "TestKonfig"() -> (w231:T5)
                    n98 = call "FGV_HovaCAL_Interface_GetData.vi"("Aktion"=Aktion_FGV_HovaCAL_Interface_GetData."reset after read", "reset index"=1) -> ()  [unwired: 5 in, 5 out]
                    n99 = call "HovaCAL Setpoints.vi"("running"=w229, "TestKonfig (Eingang)"=w231) -> ("TestKonfig (Ausgang)"=w230:T5)  [unwired: 9 in]
                    n100 = call "Konfig changes.vi"("TestKonfig alt"=w231, "TestKonfig (Eingang)"=w230) -> ("TestKonfig (Ausgang)"=w227:T5, "changed"=w228:bool)  [unwired: 4 in, 4 out]
                    n101 = case shown="True" w228 {
                      tunnel: w227 -> [_ w234]
                      frame False {
                      }
                      frame True {
                        n102 = call "FGV Interference.vi"("TestKonfig"=w234, "Aktion FGV Interference"=Aktion_FGV_Interference."TestKonfig") -> ()  [unwired: 8 in, 6 out]
                      }
                    }
                    n103 = local write "TestKonfig"(w227) -> ()
                  }
                }
              }
              frame Enabled {
                # "HovaCAL Solwerte werdenjetzt afu eigener Register Karte angezeigt, und nicht mehr \nin den Settings überschreiben ... \n\nReset der Flags jetzt wieder nur für LIN ... sonst müsste man überhaupt durchgängig 2 Flags machen ?\nEventuell die LIN irgendawn auch so umbauen ?"
              }
            }
          }
          frame "Test" {
            n104 = case shown="True" w237 {
              tunnel: w236 -> [_ w243]
              tunnel: [_ w242] -> _
              tunnel: [_ w241] -> _
              tunnel: [_ w240] -> _
              tunnel: [_ w239] -> _
              tunnel: [_ w238] -> _
              frame False {
              }
              frame True {
                n105 = call "Graph TestRun.vi"() -> ("Graph"=→"Graph" →"Graph PDF":waveform(dbl)[], "Messwerte"=w248:dbl[])  [unwired: 7 in, 3 out]
                n106 = Index Array(array=w248) -> (element #1=→"Komponentenwert":dbl, element #2=→"Referenzinterferentwert":dbl, element #3=→"Kontrollinterferentwert":dbl, element #4=→"Referenzwert":dbl)  [unwired: 4 in]
                n107 = for {
                  tunnel: w243 -> [w256] mode=indexing
                  tunnel: [w253] -> w242 mode=indexing
                  tunnel: [w251] -> w241 mode=indexing
                  tunnel: [w254] -> w240 mode=indexing
                  tunnel: [w252] -> w239 mode=indexing
                  tunnel: [w250] -> w238 mode=indexing
                  n108 = property on="Eigenschaftsknoten" class="SVDiagr (strikt)"(reference=w256) -> ("XScale.Maximum"=w253:dbl, "XScale.Minimum"=w251:dbl, "History Data"=w255:waveform(dbl)[][])  [unwired: 1 in, 2 out]
                  n109 = Array Size(array=w255) -> (size(s)=w254:i32[])
                  n110 = Seconds To Date/Time(time stamp (now)=w253) -> (date time rec=w252:T44)  [unwired: 1 in]
                  n111 = Seconds To Date/Time(time stamp (now)=w251) -> (date time rec=w250:T44)  [unwired: 1 in]
                }
              }
            }
          }
          frame "HovaCAL Status" {
            n112 = call "HovaCAL TestRun Values.vi"() -> ("Cluster.PumpModeGeneral-Cluster"=→"Cluster.PumpModeGeneral-Cluster":T20, "MFC Output"=→"MFC Output":T21, "Cluster.Temp Cluster"=→"Cluster.Temp Cluster":T45, "Water-Cluster out"=→"Pumpe":cluster{"water conc SP":dbl, "water conc":dbl}, "MFC Output Array"=w261:T23[])  [unwired: 7 in]
            n113 = Index Array(array=w261) -> (element #1=→"MFC1 Output":T23, element #2=→"MFC2 Output":T23, element #3=→"MFC3 Output":T23)  [unwired: 3 in]
          }
          frame "Result" {
          }
        }
        n114 = case shown="True" w140 {
          tunnel: [w171 w182] -> w138
          tunnel: w136 -> [w172 _]
          tunnel: w135 -> [w175 _]
          tunnel: w134 -> [w174 _]
          frame False {
            n115 = Not Equal?(x=w174, y=w175) -> (x != y?=w173:bool)
            n116 = Select(t=FALSE, s=w173, f=w172) -> (s? t:f=w171:bool)
          }
          frame True {
            # "init HovaCAL controls only once or when connection changed ..."
            n117 = disable-structure shown="TestRun==TRUE" {
              disable-tunnel: [w200 w206] -> w181
              frame condition #0 (active) {
                n118 = call "TestRun HovaCAL SystemValues.vi"() -> ("Info Cluster"=w199:T46)  [unwired: 11 in]
                n119 = stacked-sequence {
                  tunnel: w199 -> [w202 w204]
                  tunnel: [w201 _] -> w200
                  frame #0 {
                    n120 = call "FGV_HovaCAL_Interface_GetData.vi"("Aktion"=Aktion_FGV_HovaCAL_Interface_GetData."SystemInfo", "System Cluster in"=w202) -> ("System Cluster out"=w201:T46)  [unwired: 5 in, 4 out]
                  }
                  frame #1 {
                    n121 = call "FGV_HovaCAL_Interface_SetData.vi"("System Cluster in"=w204, "Aktion"=Aktion_FGV_HovaCAL_Interface_SetData."init") -> ()  [unwired: 7 in, 7 out]
                  }
                }
              }
              frame condition #1 {
                n122 = call "FGV_HovaCAL_Interface_GetData.vi"("Aktion"=Aktion_FGV_HovaCAL_Interface_GetData."lesen") -> ("System Cluster out"=w206:T46)  [unwired: 6 in, 4 out]
              }
            }
            n123 = Unbundle By Name(w181) -> ("device"=w180:string, "number of mfc"=w179:i32)
            n124 = Empty String/Path?(string/path=w180) -> (empty?=w178:bool)
            n125 = Less Than 0?(x=w179) -> (x < 0?=w177:bool)
            n126 = Or(x=w178, y=w177) -> (x .or. y?=w176:bool)
            n127 = case shown="False" w176 {
              tunnel: [TRUE ("t") _] -> w182
              tunnel: w181 -> [w183 _]
              frame False {
                # "#HovaCAL_Interference_BugFixes"
                # "Werte HovaVAL wieder setzen ... !"
                # "#HovaCAL_Interference_BugFixes"
                n128 = control-ref of="Cluster.PumpModeGeneral-Cluster"() -> (w195:refnum<vi>)
                n129 = control-ref of="HovaCAL Temperature"() -> (w198:refnum<vi>)
                n130 = control-ref of="Cluster.Temp Cluster"() -> (w197:refnum<vi>)
                n131 = control-ref of="MFC2"() -> (w194:refnum<vi>)
                n132 = control-ref of="MFC3"() -> (w193:refnum<vi>)
                n133 = Build Array(w194, w193) -> (w192:refnum<vi>[])
                n134 = Bundle("HovaCAL Temperature"=w198, "Cluster.Temp Cluster"=w197, "Cluster.PumpModeGeneral-Cluster"=w195, w192) -> (w196:T47)  [unwired: 1 in]
                n135 = call "Init_HovaCAL Controls.vi"("Refs Cluster"=w196, "Info Cluster"=w183) -> ("Fehler (Ausgang)"=w190:errorcluster)  [unwired: 9 in]
                n136 = call "FGV Interference.vi"("error in (no error)"=w190, "Aktion FGV Interference"=Aktion_FGV_Interference."Lesen") -> ("TestKonfig"=w187:T5, "error out"=w185:errorcluster)  [unwired: 8 in, 4 out]
                n137 = call "MFC verriegeln.vi"("init"=TRUE, "Fehler (Eingang, kein Fehler)"=w185, "TestKonfig (Eingang)"=w187) -> ("Fehler (Ausgang)"=w184:errorcluster, "TestKonfig (Ausgang)"=w186:T5)  [unwired: 6 in, 1 out]
                n138 = call "HovaCAL set params konfig.vi"("Fehler (Eingang, kein Fehler)"=w184, "TestKonfig (Eingang)"=w186) -> ()  [unwired: 8 in, 2 out]
              }
              frame True {
              }
            }
          }
        }
        n139 = case shown="True" w157 {
          selector: w157 -> [_ w208]
          frame False {
          }
          frame True {
            n140 = property on="Systemeinstellung" class="Bool. (strikt)"("Val(Sgnl)"=w208) -> (error out=w209:errorcluster)  [unwired: 2 in, 1 out]
            n141 = call <vilib>:"Clear Errors.vi"("error in (no error)"=w209) -> ()  [unwired: 5 in, 2 out]
          }
        }
        n142 = case shown="True" w159 {
          frame False {
          }
          frame True {
            n143 = property on="Gasliste vergleichen" class="Bool."("Val(Sgnl)"=TRUE) -> (error out=w211:errorcluster)  [unwired: 2 in, 1 out]
            n144 = call <vilib>:"Clear Errors.vi"("error in (no error)"=w211) -> ("error out"=w210:errorcluster)  [unwired: 5 in, 1 out]
            n145 = flat-sequence {
              tunnel: w210 -> [_]
              frame #0 {
              }
            }
          }
        }
        n146 = Not(x=w145) -> (.not. x?=w144:bool)
        n147 = Empty String/Path?(string/path=w166) -> (empty?=w167:bool)
        n148 = Equal?(x=w130, y=w131) -> (x = y?=w132:bool)
        n149 = Or(x=w132, y=w167) -> (x .or. y?=w133:bool)
        n150 = Select(t=T30."Enabled" ("Deaktiviert"), s=w144, f=T30."Disabled and Grayed Out" ("Deaktiviert")) -> (s? t:f=w149:T30)
        n151 = Select(t=T30."Enabled" ("Deaktiviert"), s=w145, f=T30."Disabled and Grayed Out" ("Deaktiviert")) -> (s? t:f=w146:T30)
        n152 = case shown="False" w133 {
          tunnel: w164 -> [w300 w303]
          tunnel: w166 -> [w302 _]
          tunnel: [w301 w303] -> w165
          frame False {
            n153 = call "Strings und Zeitstempel verknuepfen.vi"("String 1 hinzufügen"=w302, "Eingagns String"=w300) -> ("Verknüpfter String"=w301:string)  [unwired: 9 in]
          }
          frame True {
          }
        }
        n154 = property on="Test Start" class="Bool."("DisabledEnum"=w149) -> (error out=w151:errorcluster)  [unwired: 2 in, 1 out]
        n155 = property on="Abbrechen" class="Bool."("DisabledEnum"=w146) -> (error out=w150:errorcluster)  [unwired: 2 in, 1 out]
        n156 = call <vilib>:"Clear Errors.vi"("error in (no error)"=w151) -> ()  [unwired: 5 in, 2 out]
        n157 = call <vilib>:"Clear Errors.vi"("error in (no error)"=w150) -> ()  [unwired: 5 in, 2 out]
        n158 = local write "Anforderung"(w134) -> ()
      }
      event Value Change {
        w314 = T48 500 items=["10"=10, "11"=11, "16"=16, "32"=32, "64"=64, "128"=128, "256"=256, "500"=500, "1000"=1000] ("Gasteiler Stufen")
        w316 = T42 4 items=["LNI", "Analog-Display", "AVL GDU", "Horiba GDC", "HovaCal", "Horiba SGD 710C"] ("Gasteiler Type")
        # "GD Type und Stufenanzahl sowie COMM vorbelegen ... laden ?!?!?"
        n159 = event-data() -> ()  [unwired: 1 in, 6 out]
        n160 = call "FGV Gasteiler.vi"("Aktionen"=Aktionen_FGV_Gasteiler_Daten."lesen") -> ("Gasteiler Daten"=w317:T49, "error out"=w308:errorcluster)  [unwired: 11 in, 6 out]
        n161 = Bundle By Name(cluster=w317, "Gasteiler"=T36 "HovaCAL", "Gasteiler Stufen"=w314, "Gasteiler Type"=w316, "Gasteiler Span Eingänge"=u16 0) -> (w311:T49)
        n162 = call "FGV Gasteiler.vi"("Gasteiler Daten"=w311, "error in (no error)"=w308, "Aktionen"=Aktionen_FGV_Gasteiler_Daten."Gasteiler Daten") -> ("Gasteiler Daten"=w309:T49, "error out"=w307:errorcluster)  [unwired: 9 in, 6 out]
        n163 = call "FGV Gasteiler.vi"("Gasteiler Daten"=w309, "error in (no error)"=w307, "Aktionen"=Aktionen_FGV_Gasteiler_Daten."speichern") -> ("error out"=w306:errorcluster)  [unwired: 9 in, 7 out]
        n164 = call "FGV Stoerungen sammeln und auswerten.vi"("Errors"=T37 {"Störung Kommunikation"=FALSE, "Pressure carrier gas"=FALSE, "Pressure diluted gas"=FALSE, "Outlet Pressure"=FALSE, "SNOX before SAIR"=FALSE, "Störung Gasteiler"=FALSE} ("Eingangs-Cluster"), "error in (no error)"=w306, "Aktion"=Aktion_FGV_Stoerungen_sammeln_und_auswerten."error") -> ("error out"=w324:errorcluster)  [unwired: 10 in, 6 out]
        n165 = call "FGV Stoerungen sammeln und auswerten.vi"("error in (no error)"=w324, "Aktion"=Aktion_FGV_Stoerungen_sammeln_und_auswerten."reset error") -> ("Errors"=w323:T37, "error out"=w322:errorcluster)  [unwired: 11 in, 5 out]
        n166 = Unbundle By Name(w323) -> ("Störung Kommunikation"=→"Störung Kommunikation":bool)
        n167 = call "FGV Gasteiler.vi"("Anforderung"="Anforderung", "error in (no error)"=w322, "Aktionen"=Aktionen_FGV_Gasteiler_Daten."Anforderung") -> ()  [unwired: 9 in, 8 out]
        "Error" <- T18 {"Pressure carrier gas"=FALSE, "Pressure diluted gas"=FALSE, "Outlet Pressure"=FALSE, "SNOX before SAIR"=FALSE} ("Error")
      }
      event Value Change {
        n168 = event-data() -> ()  [unwired: 1 in, 6 out]
        n169 = call "FGV Gasteiler.vi"("Aktionen"=Aktionen_FGV_Gasteiler_Daten."lesen") -> ("Gasteiler Daten"=w349:T49)  [unwired: 11 in, 7 out]
        n170 = Unbundle By Name(w349) -> ("Gasteiler Stufen"=w348:T48)
        n171 = call "FGV Interference.vi"("Aktion FGV Interference"=Aktion_FGV_Interference."Lesen") -> ("TestKonfig"=w335:T5)  [unwired: 9 in, 5 out]
        n172 = Unbundle By Name(w335) -> ("TestKonfig H2O.Punkte umkehren"=w351:bool, "TestKonfig H2O.Anzahl Stufen"=w352:sgl)  [unwired: 1 out]
        n173 = call "Komponentenauswahl.vi"("TestKonfig in"=w335) -> ("Array"=w334:T51)  [unwired: 7 in, 3 out]
        n174 = Index Array(array=w334, index=1 ("Index")) -> (element=w339:T52)
        n175 = call "HovaCal Stufen aufteilen.vi"("Komponentenauswahl"=w339, "Punkte umkehren"=w351, "Anzahl Stufen"=w352, "Gasteiler Stufen"=w348) -> (1:"Stufen"=w345:dbl[], 3:"Stufen"=w346:u16[])  [unwired: 4 in, 2 out]
        n176 = Number To Fractional String(number=w345, precision (6)=i16 2 ("Genauigkeit (6)")) -> (F-format string=w342:string[])  [unwired: 2 in]
        n177 = Number To Decimal String(number=w346) -> (decimal integer string=w343:string[])  [unwired: 1 in]
        n178 = Build Array(w343, w342) -> (w344:string[][])
        n179 = Transpose 2D Array(2D array=w344) -> (transposed array=w338:string[][])
        n180 = Bundle By Name(cluster=w335, "TestKonfig H2O.Stufen Tabelle"=w338) -> (w340:T5)
        n181 = call "FGV Interference.vi"("TestKonfig"=w340, "Aktion FGV Interference"=Aktion_FGV_Interference."TestKonfig") -> ("error out"=w337:errorcluster)  [unwired: 8 in, 5 out]
        n182 = property on="Stufen Tabelle" class="Tbl (strikt)"(error in=w337, "Value"=w338) -> (error out=w336:errorcluster)  [unwired: 1 in, 1 out]
        n183 = call <vilib>:"Clear Errors.vi"("error in (no error)"=w336) -> ()  [unwired: 5 in, 2 out]
      }
      event "Systemeinstellung": Value Change {
        n184 = event-data() -> ()  [unwired: 1 in, 6 out]
        n185 = stacked-sequence {
          tunnel: w362 -> [_ _ _ _]
          tunnel: [_ _ _ FALSE ("start Test")] -> w361
          tunnel: w360 -> [_ w368 _ _]
          tunnel: w359 -> [_ _ w370 _]
          frame #0 {
          }
          frame #1 {
            n186 = Index Array(array=w368) -> (element #1=w367:refnum<vi>, element #2=w366:refnum<vi>)  [unwired: 2 in]
            n187 = call "Init GFauswahl.vi"("GF MFC3 (Eingang)"=w366, "GF MFC2 (Eingang)"=w367) -> ()  [unwired: 7 in, 3 out]
            n188 = control-ref of="Analysator"() -> (w369:refnum<vi>)
            n189 = call "Analysator initialisieren.vi"("Referenz Analysator"=w369) -> ()  [unwired: 9 in, 2 out]
          }
          frame #2 {
            n190 = call "Wertaenderung Systemeinstellungen.vi"("Aktion"=Aktion_Wertaenderung_Gasliste."HovaCAL Interference inaktiv") -> ()  [unwired: 13 in, 2 out]
            n191 = local write "Systemeinstellung"(FALSE ("Systemeinstellung")) -> ()
            n192 = call "Texte in VIs uebersetzen.vi"("Sprachliste"=w370, "String zum Übersetzen"="Systemeinstellungen wurden geändert.\nBitte überprüfen." ("Nachricht")) -> ("String zum Übersetzen"=w371:string)  [unwired: 9 in, 4 out]
            n193 = One Button Dialog(message=w371, button name ("OK")="OK" ("Schaltflächentext (\"OK\")")) -> ()  [unwired: 1 out]
          }
          frame #3 {
            n194 = call "FGV Interference.vi"("Aktion FGV Interference"=Aktion_FGV_Interference."Lesen") -> ("TestKonfig"=w376:T5, "error out"=w377:errorcluster)  [unwired: 9 in, 4 out]
            n195 = property on="TestKonfig" class="Cluster (strikt)"(error in=w377, "Val(Sgnl)"=w376) -> (error out=w380:errorcluster)  [unwired: 1 in, 1 out]
            n196 = call <vilib>:"Clear Errors.vi"("error in (no error)"=w380) -> ()  [unwired: 5 in, 2 out]
          }
        }
      }
      event Value Change {
        n197 = event-data() -> ()  [unwired: 1 in, 1 out]
        n198 = call "FGV Interference.vi"("TestSetting"="TestSetting", "Aktion FGV Interference"=Aktion_FGV_Interference."TestSetting") -> ("error out"=w383:errorcluster)  [unwired: 8 in, 5 out]
        n199 = call "FGV Interference.vi"("error in (no error)"=w383, "Aktion FGV Interference"=Aktion_FGV_Interference."Speichern") -> ()  [unwired: 8 in, 6 out]
      }
      event Value Change {
        w391 = 0  # Pump Idx
        # "Pumpe Index 0 passt für alle HovaCAL ?!"
        # "Stufenanzahl geändert  ... neu Abfragen ?!?!"
        n200 = event-data() -> ()  [unwired: 1 in, 6 out]
        n201 = call "FGV Interference.vi"("Aktion FGV Interference"=Aktion_FGV_Interference."Lesen") -> ("TestKonfig"=w421:T5, "error out"=w418:errorcluster)  [unwired: 9 in, 4 out]
        n202 = call "Gasflaschen Aenderung.vi"("init"=FALSE, "Fehler (Eingang, kein Fehler)"=w418, "TestKonfig alt"=w421, "TestKonfig (Eingang)"="TestKonfig") -> ("Fehler (Ausgang)"=w422:errorcluster, "TestKonfig alt out"=w420:T5, "TestKonfig (Ausgang)"=w423:T5)  [unwired: 5 in]
        n203 = call "MFC verriegeln.vi"("init"=FALSE, "Fehler (Eingang, kein Fehler)"=w422, "TestKonfig alt (Eingang)"=w420, "TestKonfig (Eingang)"=w423) -> ("Fehler (Ausgang)"=w399:errorcluster, "TestKonfig alt (Eingang) out"=w400:T5, "TestKonfig (Ausgang)"=w401:T5)  [unwired: 5 in]
        n204 = call "HovaCAL Stufentabelle aendern.vi"("Fehler (Eingang, kein Fehler)"=w399, "TestKonfig alt"=w400, "TestKonfig (Eingang)"=w401) -> ("Fehler (Ausgang)"=w398:errorcluster, "TestKonfig (Ausgang)"=w397:T5)  [unwired: 7 in]
        n205 = call "FGV Interference.vi"("TestKonfig"=w397, "error in (no error)"=w398, "Aktion FGV Interference"=Aktion_FGV_Interference."TestKonfig") -> ("TestKonfig"=w396:T5, "error out"=w395:errorcluster)  [unwired: 7 in, 4 out]
        n206 = call "HovaCAL set params konfig.vi"("Fehler (Eingang, kein Fehler)"=w395, "Pump Idx"=w391, "TestKonfig (Eingang)"=w396) -> ("Fehler (Ausgang)"=w394:errorcluster, "TestKonfig (Ausgang)"=w393:T5)  [unwired: 7 in]
        n207 = call "Initialisieren.vi"("MFC Cluster Array"=w392, "TestKonfig (Eingang)"=w393, "Fehler (Eingang)"=w394, "Strings Array in"=w437, "Ergebnis  Array in"=w438, "Signalverlaufsdiagramm (Eingang)"=w426) -> ("Fehler (Ausgang)"=w429:errorcluster, "Ergenis Arry out"=w433:refnum<vi>[])  [unwired: 2 in, 2 out]
        n208 = call "Index uebersetzen.vi"("Aktion"=Aktion_Index_uebersetzten."auswerten", "error in (no error)"=w429) -> ("error out"=w404:errorcluster, "Komponenten"=w402:T28)  [unwired: 4 in, 4 out]
        n209 = Unbundle By Name(w402) -> ("Komponente"=→"Komponente 1S:":T15, "Referenz Interferent"=→"Interferent 1:" →"Referenzwert:":T15, "Kontroll Interferent"=→"Interferent 2:":T15)
        n210 = Unbundle By Name(w402) -> ("Einheit Komponente"=w408:string, "Einheit Refernz Interferrent"=w407:string, "Einheit Kontroll Interferrent"=w406:string)
        n211 = Build Array(w408, w407, w406) -> (w405:string[])
        n212 = call "FGV Interference.vi"("Einheiten"=w405, "error in (no error)"=w404, "Aktion FGV Interference"=Aktion_FGV_Interference."Einheiten") -> ("error out"=w403:errorcluster)  [unwired: 7 in, 5 out]
        n213 = call "Init Einheiten.vi"("TestKonfig (Eingang)"=w393, "Units Array in"=w416, "Fehler (Eingang, kein Fehler)"=w403, "Komp. Auswahl Array"=w436, "Ergebnis Array in"=w433, "Table Array in"=w415) -> ("Fehler (Ausgang)"=w432:errorcluster)  [unwired: 5 out]
        n214 = call <vilib>:"Clear Errors.vi"("error in (no error)"=w432) -> ("error out"=w430:errorcluster)  [unwired: 5 in, 1 out]
        n215 = call "Wertaenderung Gasliste.vi"("error in (no error)"=w430, "Aktion"=Aktion_Wertaenderung_Gasliste."HovaCAL Interference inaktiv") -> ("error out"=w427:errorcluster)  [unwired: 12 in, 1 out]
        n216 = call "FGV Interference.vi"("error in (no error)"=w427, "Aktion FGV Interference"=Aktion_FGV_Interference."Speichern") -> ("TestKonfig"=w424:T5)  [unwired: 8 in, 5 out]
        n217 = local write "TestKonfig"(w424) -> ()
      }
      event "Gasliste vergleichen": Value Change {
        n218 = event-data() -> ()  [unwired: 1 in, 6 out]
        n219 = call "FGV Interference.vi"("Aktion FGV Interference"=Aktion_FGV_Interference."Lesen") -> ("TestKonfig"=w456:T5, "error out"=w457:errorcluster)  [unwired: 9 in, 4 out]
        n220 = Index Array(array=w450) -> (element #1=w474:refnum<vi>, element #2=w473:refnum<vi>, element #3=w472:refnum<vi>)  [unwired: 3 in]
        n221 = call "Init Komponentenauswahl.vi"("Fehler (Eingang, kein Fehler)"=w457, "Kontroll-Interferent: (Eingang)"=w472, "Refernz-Interferent: (Eingang)"=w473, "Komponente: (Eingang)"=w474) -> ("Fehler (Ausgang)"=w459:errorcluster, "Komponenten"=w455:T28)  [unwired: 3 in, 3 out]
        n222 = Unbundle By Name(w455) -> ("Einheit Komponente"=w464:string, "Einheit Refernz Interferrent"=w463:string, "Einheit Kontroll Interferrent"=w462:string)
        n223 = call "Gasflaschen Aenderung.vi"("init"=TRUE, "Fehler (Eingang, kein Fehler)"=w459, "TestKonfig alt"=w456, "TestKonfig (Eingang)"=w456) -> ("Fehler (Ausgang)"=w467:errorcluster, "TestKonfig alt out"=w468:T5, "TestKonfig (Ausgang)"=w469:T5)  [unwired: 5 in]
        n224 = call "MFC verriegeln.vi"("init"=TRUE, "Fehler (Eingang, kein Fehler)"=w467, "TestKonfig alt (Eingang)"=w468, "TestKonfig (Eingang)"=w469) -> ("Fehler (Ausgang)"=w460:errorcluster, "TestKonfig (Ausgang)"=w466:T5)  [unwired: 5 in, 1 out]
        n225 = Build Array(w464, w463, w462) -> (w461:string[])
        n226 = call "FGV Interference.vi"("Einheiten"=w461, "error in (no error)"=w460, "Aktion FGV Interference"=Aktion_FGV_Interference."Einheiten") -> ("error out"=w454:errorcluster)  [unwired: 7 in, 5 out]
        n227 = call "Texte in VIs uebersetzen.vi"("Sprachliste"=w443, "String zum Übersetzen"="Gasliste wurde geändert.\nBitte überprüfen." ("Nachricht")) -> ("String zum Übersetzen"=w444:string)  [unwired: 9 in, 4 out]
        n228 = call "Init Einheiten.vi"("TestKonfig (Eingang)"=w466, "Units Array in"=w453, "Fehler (Eingang, kein Fehler)"=w454, "Komp. Auswahl Array"=w450, "Ergebnis Array in"=w451, "Table Array in"=w452) -> ("Fehler (Ausgang)"=w449:errorcluster, "TestKonfig (Ausgang)"=w448:T5)  [unwired: 4 out]
        n229 = One Button Dialog(message=w444, button name ("OK")="OK" ("Schaltflächentext (\"OK\")")) -> ()  [unwired: 1 out]
        n230 = property on="TestKonfig" class="Cluster (strikt)"(error in=w449, "Val(Sgnl)"=w448) -> (error out=w447:errorcluster)  [unwired: 1 in, 1 out]
        n231 = call <vilib>:"Clear Errors.vi"("error in (no error)"=w447) -> ()  [unwired: 5 in, 2 out]
      }
      event "Test Start": Value Change {
        n232 = event-data() -> ()  [unwired: 1 in, 6 out]
        n233 = call "Test Status.vi"("Aktion"=Aktion_Test_Status."lesen") -> ("Tests sperren"=w485:bool)  [unwired: 11 in, 3 out]
        n234 = call "Test HovaCAL Start Kondition.vi"("Sprachliste"=w489) -> ("ok"=w487:bool)  [unwired: 9 in, 1 out]
        n235 = Not(x=w487) -> (.not. x?=w486:bool)
        n236 = Or(x=w485, y=w486) -> (x .or. y?=w488:bool)
        n237 = case shown="False" w488 {
          tunnel: [w520 FALSE] -> w493
          tunnel: w489 -> [w501 w537]
          tunnel: [w518 w536] -> w491
          tunnel: w490 -> [w517 w536]
          tunnel: w485 -> [_ w535]
          tunnel: w483 -> [w510 _]
          tunnel: w482 -> [w508 _]
          tunnel: ["" _] -> w481
          tunnel: w479 -> [w495 _]
          tunnel: [w494 _] -> _
          frame False {
            w505 = T42 4 items=["LNI", "Analog-Display", "AVL GDU", "Horiba GDC", "HovaCal", "Horiba SGD 710C"] ("x")
            w516 = 0  # Pump Idx
            # "Pumpe Index 0 passt für alle HovaCAL ?!"
            # "HovaCAL aktiv ?\nTemp. erreicht ? Flow Setpoint > 0 ?\nIn LIN setzen ?!"
            n238 = call "FGV Gasteiler.vi"("Aktionen"=Aktionen_FGV_Gasteiler_Daten."lesen") -> ("Gasteiler Type"=w506:T42, "Anforderung"=w502:bool)  [unwired: 11 in, 6 out]
            n239 = Equal?(x=w505, y=w506) -> (x = y?=w504:bool)
            n240 = call "Graph loeschen.vi"("Ergebnis  Array in"=w508, "Graph"=w510) -> ("Fehler (Ausgang)"=w509:errorcluster, "Graph out"=w496:refnum<vi>[])  [unwired: 7 in, 1 out]
            n241 = And(x=w504, y=w502) -> (x .and. y?=w503:bool)
            n242 = call "FGV Interference.vi"("error in (no error)"=w509, "Aktion FGV Interference"=Aktion_FGV_Interference."Lesen") -> ("TestKonfig"=w500:T5, "error out"=w498:errorcluster)  [unwired: 8 in, 4 out]
            n243 = case shown="False" w503 {
              tunnel: w502 -> [w524 _]
              tunnel: w501 -> [w523 _]
              frame False {
                n244 = case shown="True" w524 {
                  tunnel: w523 -> [w525 w529]
                  frame False {
                    # "keine Anforderung GD"
                    n245 = call "Texte in VIs uebersetzen.vi"("Sprachliste"=w525, "String zum Übersetzen"="Keine Verbindung zum Gasteiler.\nBitte überprüfen." ("Nachricht")) -> ("String zum Übersetzen"=w526:string)  [unwired: 9 in, 4 out]
                    n246 = One Button Dialog(message=w526, button name ("OK")="OK" ("Schaltflächentext (\"OK\")")) -> ()  [unwired: 1 out]
                  }
                  frame True {
                    # "GD Type nicht HovaCAL"
                    n247 = call "Texte in VIs uebersetzen.vi"("Sprachliste"=w529, "String zum Übersetzen"="Ausgewählte Gasteiler Type ist nicht HovaCAL.\nBitte überprüfen." ("Nachricht")) -> ("String zum Übersetzen"=w530:string)  [unwired: 9 in, 4 out]
                    n248 = One Button Dialog(message=w530, button name ("OK")="OK" ("Schaltflächentext (\"OK\")")) -> ()  [unwired: 1 out]
                  }
                }
              }
              frame True {
              }
            }
            n249 = call "Graph Max Points.vi"("Fehler (Eingang, kein Fehler)"=w498, "Spülen"=w495, "Signalverlaufsdiagramm (Eingang)"=w496, "TestKonfig in"=w500) -> ("Fehler (Ausgang)"=w497:errorcluster, "Max. Wert out"=w494:dbl, "TestKonfig out"=w499:T5)  [unwired: 4 in, 1 out]
            n250 = Unbundle By Name(w499) -> ("TestKonfig H2O.Anzahl Stufen"=w511:sgl)
            n251 = disable-structure shown="TestRun==FALSE, Standard" {
              disable-tunnel: [FALSE TRUE] -> w521
              frame condition #0 {
              }
              frame condition #1 (active) {
              }
            }
            n252 = call "LIN Parameter setzen für Aufzeichnung und Auswertung.vi"("Fehler (Eingang, kein Fehler)"=w497, "TestKonfig in"=w499) -> ("Fehler (Ausgang)"=w512:errorcluster, "TestKonfig out"=w513:T5)  [unwired: 8 in]
            n253 = Or(x=w521, y=w503) -> (x .or. y?=w520:bool)
            n254 = call "HovaCAL set params on start.vi"("Fehler (Eingang, kein Fehler)"=w512, "Pump Idx"=w516, "TestKonfig (Eingang)"=w513) -> ("Fehler (Ausgang)"=w514:errorcluster)  [unwired: 7 in, 1 out]
            n255 = Select(t=Aktion_Test."ini" ("Aktion"), s=w520, f=w517) -> (s? t:f=w518:T24)
            n256 = call "HovaCAL fix Sollwerte in Tabelle.vi"("error in (no error)"=w514, "Anzahl Stufen"=w511) -> ()  [unwired: 9 in, 1 out]
          }
          frame True {
            n257 = case shown="False" w535 {
              tunnel: w537 -> [w539 w543]
              frame True {
                n258 = call "Texte in VIs uebersetzen.vi"("Sprachliste"=w539, "String zum Übersetzen"="Anderer Test läuft gerade.\nBitte etwas Geduld." ("Nachricht")) -> ("String zum Übersetzen"=w540:string)  [unwired: 9 in, 4 out]
                n259 = One Button Dialog(message=w540, button name ("OK")="OK" ("Schaltflächentext (\"OK\")")) -> ()  [unwired: 1 out]
              }
              frame False {
                n260 = call "Texte in VIs uebersetzen.vi"("Sprachliste"=w543, "String zum Übersetzen"="HovaCAL Startbedingungen nicht erfüllt.\nBitte überprüfen." ("Nachricht")) -> ("String zum Übersetzen"=w544:string)  [unwired: 9 in, 4 out]
                n261 = One Button Dialog(message=w544, button name ("OK")="OK" ("Schaltflächentext (\"OK\")")) -> ()  [unwired: 1 out]
              }
            }
          }
        }
      }
      event "Abbrechen": Value Change {
        n262 = event-data() -> ()  [unwired: 1 in, 3 out]
        n263 = call "Test Status.vi"("Aktion"=Aktion_Test_Status."lesen") -> ("Aktive Tests"=w552:T43, "Tests sperren"=w550:bool)  [unwired: 11 in, 2 out]
        n264 = Unbundle By Name(w552) -> ("HovaCAL Interference läuft"=w551:bool)
        n265 = And(x=w551, y=w550) -> (x .and. y?=w549:bool)
        n266 = case shown="True" w549 {
          tunnel: [w559 w564] -> w558
          tunnel: w557 -> [w559 w563]
          tunnel: w554 -> [_ w560]
          frame False {
          }
          frame True {
            n267 = call "Texte in VIs uebersetzen.vi"("Sprachliste"=w560, "String zum Übersetzen"="Test abgebrochen" ("String 1 hinzufügen")) -> ("String zum Übersetzen"=w561:string)  [unwired: 9 in, 4 out]
            n268 = call "Strings und Zeitstempel verknuepfen.vi"("String 1 hinzufügen"=w561, "Eingagns String"=w563) -> ("Verknüpfter String"=w564:string)  [unwired: 9 in]
          }
        }
      }
      event "Daten löschen": Value Change {
        n269 = event-data() -> ()  [unwired: 1 in, 3 out]
        n270 = call "FGV Interference.vi"("Aktion FGV Interference"=Aktion_FGV_Interference."löschen") -> ("Tabelle"=w567:T15[][])  [unwired: 9 in, 5 out]
        n271 = local write "Komponente"(w567) -> ()
        n272 = local write "Kontroll Interferent"(w567) -> ()
        n273 = local write "Referenz Interferent"(w567) -> ()
      }
      event "Print to PDF": Value Change {
        n274 = event-data() -> ()  [unwired: 1 in, 1 out]
        n275 = Index Array(array=w578) -> (element #2=w577:refnum<vi>)  [unwired: 2 in, 1 out]
        n276 = call "FGV Interference.vi"("Aktion FGV Interference"=Aktion_FGV_Interference."Lesen") -> ("TestSetting"=w588:T2)  [unwired: 9 in, 5 out]
        n277 = Unbundle By Name(w588) -> ("Pfad:"=w587:path, "Textname:"=w575:string)
        n278 = call "Dateiname mit Zeitstempel.vi"("Extension in"=".pdf", "File Name in"=w575) -> ("File Name"=w573:string)  [unwired: 9 in]
        n279 = Build Path(base path=w587, name or relative path=w573) -> (appended path=w579:path)
        n280 = disable-structure shown="BullZip==TRUE" {
          disable-tunnel: w579 -> [w600 _]
          disable-tunnel: [w599 _] -> w581
          frame condition #0 {
            n281 = call "Save to PDF File using BullZip 2009.vi"("Save PDF File Path"=w600) -> ("error out"=w599:errorcluster)  [unwired: 10 in]
          }
          frame condition #1 (active) {
          }
        }
        n282 = disable-structure shown="Aktiviert" {
          disable-tunnel: w581 -> [_ w596]
          disable-tunnel: [_ w595] -> w580
          disable-tunnel: w579 -> [_ w594]
          disable-tunnel: w577 -> [_ w593]
          frame Disabled {
          }
          frame Enabled {
            # "#PDF_Interface"
            n283 = call "PDF_Interface_PDF Protokoll EPA1065_InterferenceVerification.vi"("error in (no error)"=w596, "Signalverlaufsdiagramm (Eingang)"=w593, "Save PDF File Path"=w594) -> ("error out"=w595:errorcluster)  [unwired: 8 in]
          }
        }
        n284 = case shown="Fehler" w580 {
          tunnel: ["Daten gespeichert!" ("String") "Fehler beim schreiben der Daten" ("String")] -> w585
          frame No Error {
          }
          frame Error {
          }
        }
        n285 = call <vilib>:"Clear Errors.vi"("error in (no error)"=w580) -> ()  [unwired: 5 in, 2 out]
        n286 = call "Tabelle in die einzelnen Seiten zerlegen.vi"("Aktion"=FGV_Aktion_Tabelle_zerlegen."vereinzeln", "Index (Seite)"=38) -> ("Sprachliste"=w584:string[][])  [unwired: 7 in, 2 out]
        n287 = call "Texte in VIs uebersetzen.vi"("Sprachliste"=w584, "String zum Übersetzen"=w585) -> ("String zum Übersetzen"=w586:string)  [unwired: 9 in, 4 out]
        n288 = One Button Dialog(message=w586) -> ()  [unwired: 1 in, 1 out]
      }
      event "Save to file": Value Change {
        n289 = event-data() -> ()  [unwired: 1 in, 1 out]
        n290 = disable-structure shown="Deaktiviert" {
          frame Disabled {
            n291 = call "FGV Interference.vi"("Aktion FGV Interference"=Aktion_FGV_Interference."Lesen") -> ("TestSetting"=w620:T2)  [unwired: 9 in, 5 out]
            n292 = Unbundle By Name(w620) -> ("Pfad:"=w619:path, "Textname:"=w618:string)
            n293 = Concatenate Strings(w618, ".txt") -> (w623:string)
            n294 = Build Path(base path=w619, name or relative path=w623) -> (appended path=w607:path)
            n295 = Open/Create/Replace File(file path (use dialog)=w607, operation (0:open)=T40."replace or create with confirmation" ("Operation (0:Öffnen)")) -> (refnum out=w609:refnum<file>, error out=w610:errorcluster)  [unwired: 4 in, 1 out]
            n296 = Write to Text File(file (use dialog)=w609, error in=w610) -> (refnum out=w612:refnum<file>, error out=w606:errorcluster)  [unwired: 2 in, 1 out]
            n297 = Close File(refnum=w612, error in=w606) -> (error out=w611:errorcluster)  [unwired: 1 out]
            n298 = call <vilib>:"Clear Errors.vi"("error in (no error)"=w611) -> ()  [unwired: 5 in, 2 out]
            n299 = case shown="Fehler" w606 {
              tunnel: ["Daten gespeichert!" ("String") "Fehler beim schreiben der Daten" ("String")] -> w616
              frame No Error {
              }
              frame Error {
              }
            }
            n300 = call "Tabelle in die einzelnen Seiten zerlegen.vi"("Aktion"=FGV_Aktion_Tabelle_zerlegen."vereinzeln", "Index (Seite)"=38) -> ("Sprachliste"=w615:string[][])  [unwired: 7 in, 2 out]
            n301 = call "Texte in VIs uebersetzen.vi"("Sprachliste"=w615, "String zum Übersetzen"=w616) -> ("String zum Übersetzen"=w617:string)  [unwired: 9 in, 4 out]
            n302 = One Button Dialog(message=w617) -> ()  [unwired: 1 in, 1 out]
          }
          frame Enabled {
          }
        }
      }
      event "Speichern": Value Change {
        n303 = event-data() -> ()  [unwired: 1 in, 6 out]
        n304 = call "FGV Interference.vi"("Aktion FGV Interference"=Aktion_FGV_Interference."Speichern") -> ()  [unwired: 9 in, 6 out]
      }
      event "Graph löschen": Value Change {
        n305 = event-data() -> ()  [unwired: 1 in, 3 out]
        n306 = call "Graph loeschen.vi"("Ergebnis  Array in"=w633, "Graph"=w634) -> ()  [unwired: 7 in, 3 out]
      }
      event "Registerkarte": Value Change {
        n307 = event-data() -> ()  [unwired: 1 in, 6 out]
        n308 = local read "Registerkarte"() -> (w640:T1)
        n309 = case shown="\"Test Settings\"" w640 {
          frame "General Settings", Default {
          }
          frame "Test Settings" {
            # "#HovaCAL_Interference_BugFixes"
            n310 = call "FGV_HovaCAL_Interface_GetData.vi"("first flags in"=T41 {"first contact in"=TRUE, "first actual values in "=TRUE}, "Aktion"=Aktion_FGV_HovaCAL_Interface_GetData."first contact") -> ()  [unwired: 5 in, 5 out]
          }
          frame "Test" {
          }
          frame "Result" {
            n311 = call "Tabellen.vi"() -> ("Tabelle Kontroll Interferent"=→"Kontroll Interferent":string[][], "Tabbelle Referenz Interferent"=→"Referenz Interferent":string[][], "Tabelle Komponente"=→"Komponente":string[][])  [unwired: 5 in, 4 out]
          }
        }
      }
    }
    "Status" <- w114
    n312 = Not Equal?(x=w116, y=w114) -> (x != y?=w115:bool)
    n313 = case shown="True" w115 {
      frame False {
      }
      frame True {
        n314 = property on="Status" class="Str"("Text.Scroll Position"=u32 9999 ("Text.Anzeigeposition")) -> (error out=w651:errorcluster)  [unwired: 2 in, 1 out]
        n315 = call <vilib>:"Clear Errors.vi"("error in (no error)"=w651) -> ()  [unwired: 5 in, 2 out]
      }
    }
  }
